vi "Auto_New.vi"() -> ()   [LabVIEW 2017]
uses:
  Control/Saurabh/prosucer_consumer_enum1.ctl
  <vilib>/Utility/error.llb/DialogType.ctl
  <vilib>/addons/database/Connection.llb/DB Tools Open Connec (String).vi
  Global/DATA LOG.vi
  Global/Global 1.vi
  <vilib>/addons/database/NI_Database_API.lvlib
panel:
  out "SHIFT":string
  in  "BARCODE RECIPE":string(combo)
  out "PLC COM.":bool
  out "SHIFT_DATA":string[](array[string])
  out "stop":bool
  out "error out 2":errorcluster
  out "Shift 4":i32
  out "Time Stamp Out":timestamp[](array[timestamp]) format="%<%X>T"
  out "Time Stamp Out 4":timestamp[](array[timestamp]) format="%<%X>T"
  out "Shift_change":bool
  out "appended array":string[][](array[string])
  out "SHIFT_DATA 2":string[](array[string])
  in  "error in (no error)":errorcluster
  in  "Tab Control":enum32{"Screen 1", "Screen 2", "Daignostic"}(tab)
  out "OP 50":bool
  out "OP 40":bool
  out "OP 30":bool
  out "OP - 50":T1 {"RH Motor Screw" format="%#.2g N-m"; "LH Motor Screw" format="%#.2g N-m"; "Nut Torque" format="%#.2g N-m"}
  out "OP - 40":T2 {"Stack Load" format="%.2f kg"; "Dispalcement" format="%#.2g mm"; "LH Screw" format="%#.2g N-m"; "RH Screw" format="%#.2g N-m"}
  out "OP - 30":T3 {"Shaft Press Load" format="%#.2g kg"; "Displacement" format="%#.2g mm"}
  in  "stop 2":bool
  out "OP - 10":T4 {"Leak Rate" format="%#.2g SCCM"}
  in  "SIMULATE INPUT":bool[](array[boolean])=[FALSE, FALSE, FALSE, FALSE]
  out "OP - 20":T5 {"Top Load" format="%#.2g kg"; "Top Displace" format="%#.2g mm"; "Bottom Load" format="%#.2g kg"; "Bottom Displace" format="%#.2g mm"}
  out "OP 10 & 20":bool
  out "OP - 60":T6 {"Screw 6" format="%#.2g N-m"; "Screw 5" format="%#.2g N-m"; "Screw 4" format="%#.2g N-m"; "Screw 3" format="%#.2g N-m"; "Screw 2" format="%#.2g N-m"; "Screw 1" format="%#.2g N-m"}
  out "OP - 70":T7 {"Full Open" format="%#.4g V"; "Full Close" format="%#.4g V"}
  out "OP - 110":cluster{"BARCODE":string}
  out "OP - 80":T8 {"Plug Press Load" format="%#.2f kg"}
  out "OP - 90":T9 {"Steam Leak" format="%#_g sccm"; "Seat Leak" format="%#_g LPM"}
  out "OP - 100":T10 {"Response Time REV" format="%#_g msec"; "Response time FWD" format="%#_g msec"; "Motor Full Open" format="%#.2f V"; "Motor Start Back" format="%#.2f V"; "Motor Full Close" format="%#.2f V"; "Motor Start Of Close" format="%#.2f V"; "Motor Peak" format="%#.2f A"; "Sensor O/P Full Close" format="%#.2f V"; "Sensor O/P Start Of Close" format="%#.2f V"; "Sensor O/P Open" format="%#.2f V"}
  out "OP 60":bool
  out "OP 70 & 80":bool
  out "OP 90 -100 - 110":bool
  out "OP110 STATUS":dbl[](array[numeric])
  out "SCAN OP110":string[](array[string])
  out "OP100 STATUS":dbl[](array[numeric])
  out "SCAN OP100":string[](array[string])
  out "OP50 STATUS":dbl[](array[numeric])
  out "SCAN OP50":string[](array[string])
  out "OP90 STATUS":dbl[](array[numeric])
  out "SCAN OP90":string[](array[string])
  out "OP80 STATUS":dbl[](array[numeric])
  out "SCAN OP80":string[](array[string])
  out "OP70 STATUS":dbl[](array[numeric])
  out "SCAN OP70":string[](array[string])
  out "OP60 STATUS":dbl[](array[numeric])
  out "SCAN OP60":string[](array[string])
  out "OP40 STATUS":dbl[](array[numeric])
  out "SCAN OP40":string[](array[string])
  out "OP30 STATUS":dbl[](array[numeric])
  out "SCAN OP30":string[](array[string])
  out "OP20 STATUS":dbl[](array[numeric])
  out "SCAN OP20":string[](array[string])
  out "OP10 STATUS":dbl[](array[numeric])
  out "SCAN OP10":string[](array[string])
  # "Op10 20\nOp30\nOp 40\nOp50\nOp60\nOp70-80\nOp 90-100-110"
  # "SENSOR MIN VLTG"
  # "OP - 50"
  # "OP - 40"
  # "OP - 30"
  # "OP - 10"
  # "OP - 20"
  # "OP - 60"
  # "OP - 70"
  # "OP - 110"
  # "OP - 80"
  # "OP - 90"
  # "OP - 100"
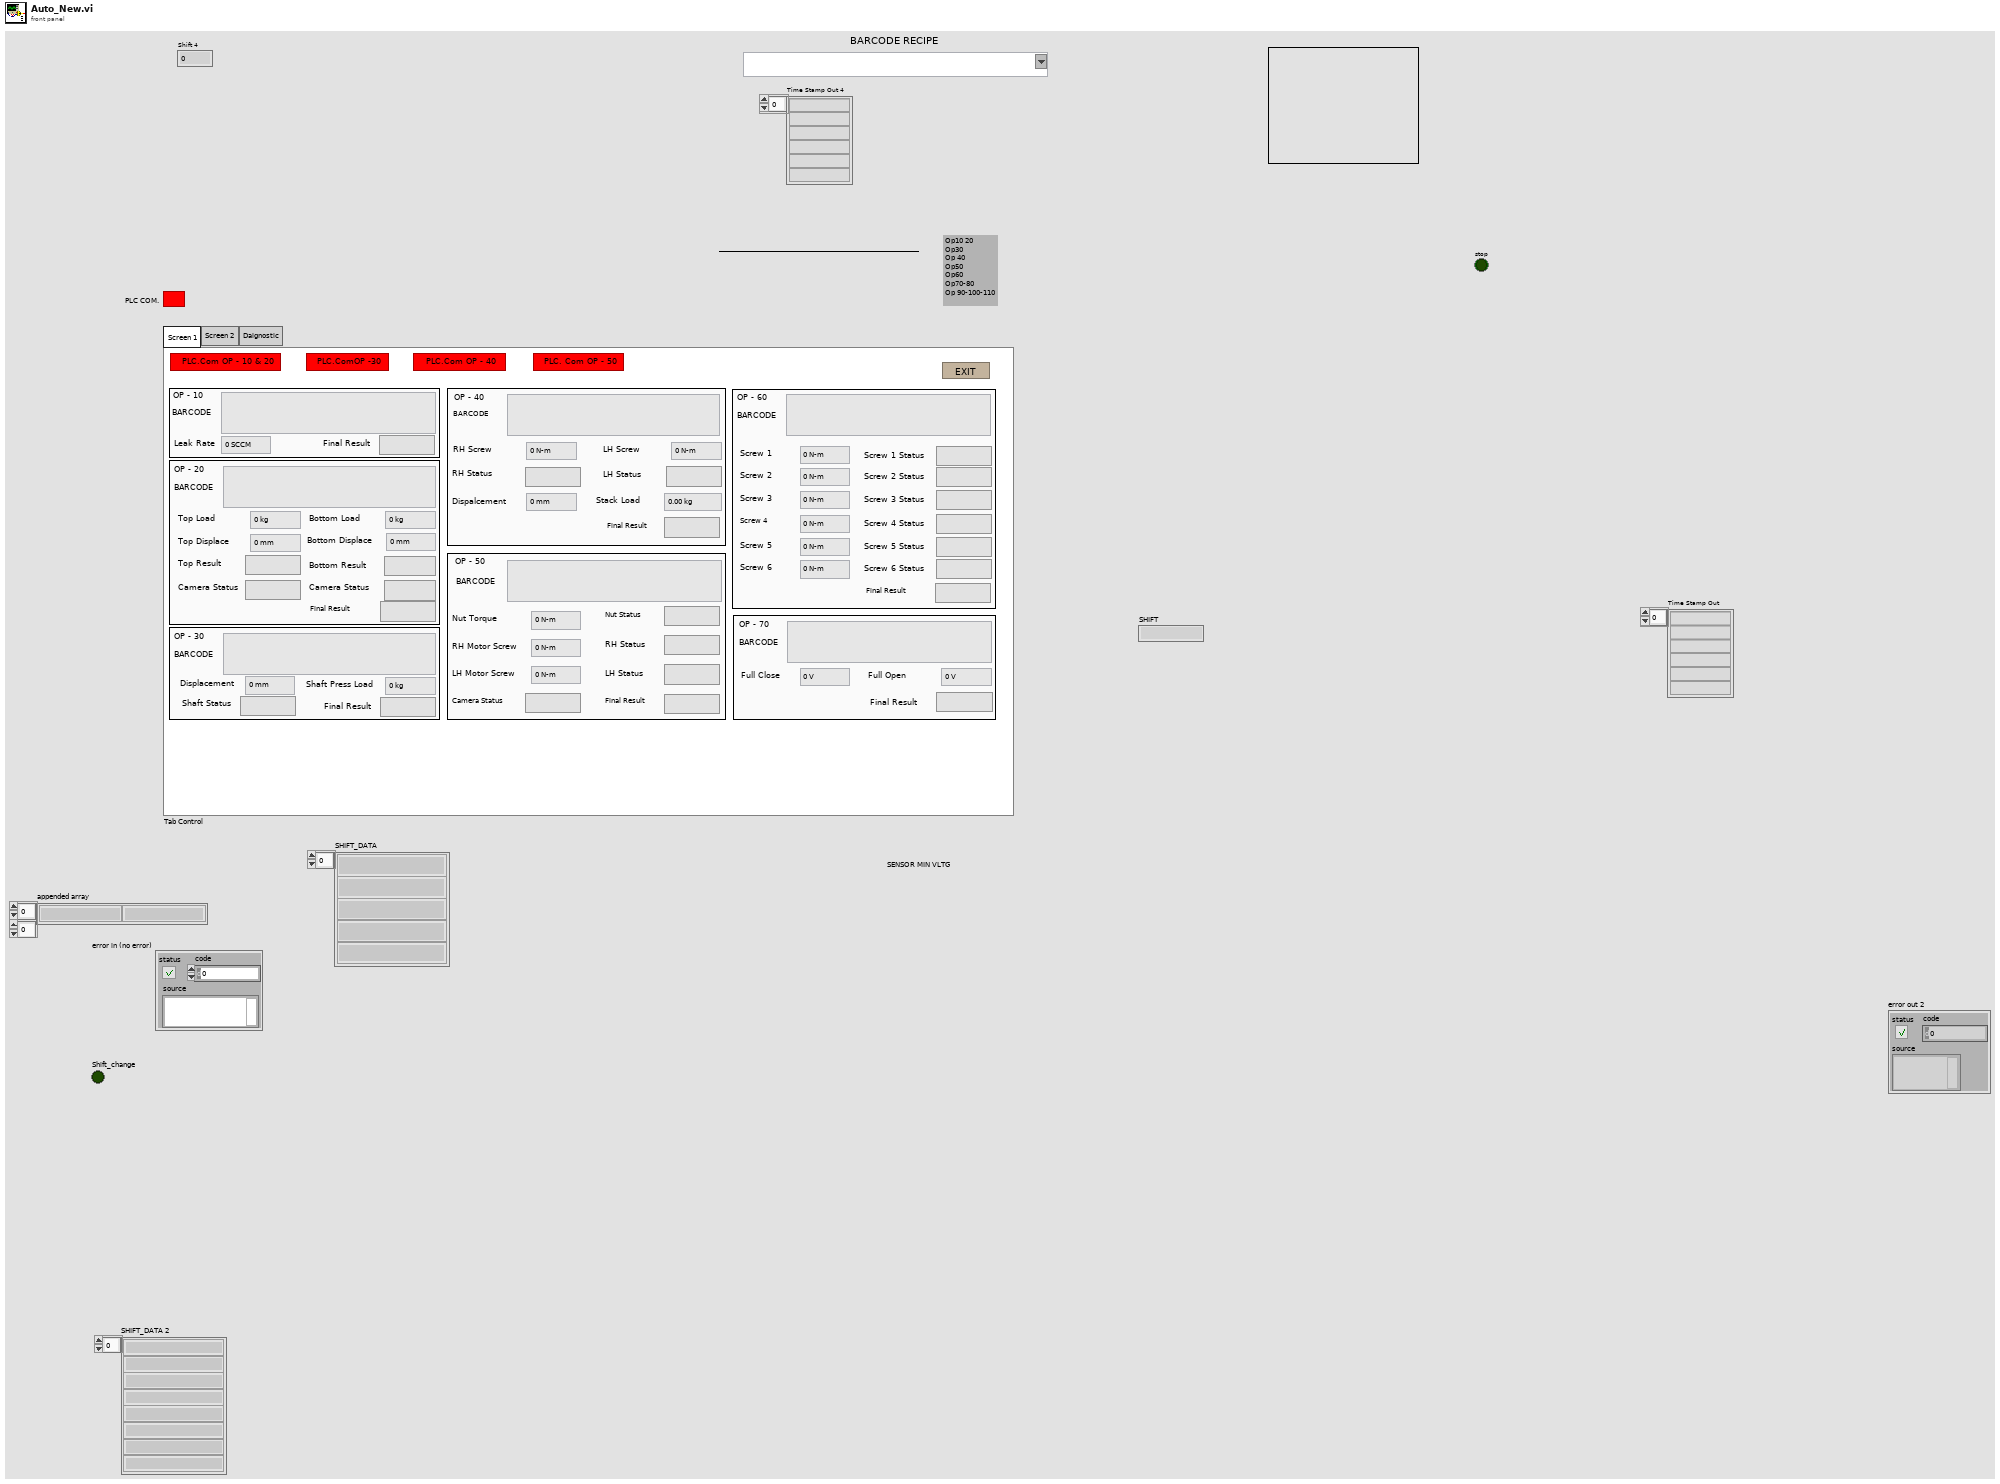
[diagram p1: front panel]
types:
  T1 = cluster{"BARCODE":string, "Nut Torque":dbl, "LH Motor Screw":dbl, "LH Status":bool, "RH Status":bool, "RH Motor Screw":dbl, "Final Result":bool, "Nut Status":bool, "Camera Status":bool}
  T2 = cluster{"BARCODE":string, "RH Screw":dbl, "LH Screw ":dbl, "RH Status":bool, "LH Status":bool, "Dispalcement ":dbl, "Stack Load ":dbl, "Final Result":bool}
  T3 = cluster{"BARCODE":string, "Displacement":dbl, "Shaft Press Load":dbl, "Shaft Status":bool, "Final Result":bool}
  T4 = cluster{"BARCODE":string, "Leak Rate":dbl, "Final Result":bool}
  T5 = cluster{"BARCODE":string, "Bottom Displace":dbl, "Bottom Load":dbl, "Camera Status":bool, "Bottom Result":bool, "Top Displace":dbl, "Top Load ":dbl, "Camera Status":bool, "Top Result":bool, "Final Result":bool}
  T6 = cluster{"BARCODE":string, "Screw 1":dbl, "Screw 2":dbl, "Screw 1 Status":bool, "Screw 2 Status":bool, "Screw 3":dbl, "Final Result":bool, "Screw 3 Status":bool, "Screw 4":dbl, "Screw 5":dbl, "Screw 4 Status":bool, "Screw 5 Status":bool, "Screw 6":dbl, "Screw 6 Status":bool}
  T7 = cluster{"BARCODE":string, "Full Close":dbl, "Full Open":dbl, "Final Result":bool}
  T8 = cluster{"BARCODE":string, "Plug Press Load":dbl, "Final Result":bool, "Loctite Status":bool}
  T9 = cluster{"BARCODE":string, "Seat Leak":dbl, "Seat Status":bool, "Steam Leak":dbl, "Final Result":bool}
  T10 = cluster{"BARCODE":string, "Sensor O/P Open":dbl, "Sensor O/P Start Of Close":dbl, "Final Result":bool, "Sensor O/P Full Close":dbl, "Motor Peak":dbl, "Motor Start Of Close":dbl, "Motor Full Close":dbl, "Motor Start Back":dbl, "Motor Full Open":dbl, "Response time FWD":dbl, "Response Time REV":dbl, "Camera Status":bool}
  T11 = cluster{"OP - 10":cluster{"BARCODE":string, "LEAK RATE":dbl, "RESULT":bool}, "OP - 30":cluster{"BARCODE":string, "Displacement":dbl, "Load":dbl, "Middle Gear Shaft Status":bool, "Final Result":bool}, "OP - 60":cluster{"BARCODE":string, "Screw 1 Data":dbl, "Screw 2 data":dbl, "Screw 1 Status":bool, "Screw 2 Status":bool, "Screw3 Data":dbl, "Final Result":bool, "Screw3 Status":bool, "Screw4 Data":dbl, "Screw5 Data":dbl, "Screw4 Status":bool, "Screw5 Status":bool, "Screw6 Data":dbl, "Screw6 Status":bool}, "OP - 70":cluster{"BARCODE":string, "Sensor MIN Vltg":dbl, "Sensor MAX Vltg":dbl, "Final Result":bool}, "OP - 80":cluster{"BARCODE":string, "Load":dbl, "Final Result":bool, "Dispensing":bool}, "OP - 90":cluster{"BARCODE":string, "Seat LT Data":dbl, "Seat Status":bool, "Steam LT Data":dbl, "Final Result":bool}, "OP - 110":cluster{"BARCODE":string}, "OP - 20":cluster{"BARCODE":string, "Bottom Displace":dbl, "Bottom Load":dbl, "Camera Status":bool, "Bottom Result":bool, "Top Displace":dbl, "Top Load ":dbl, "Camera Status":bool, "Top Result":bool, "Final Result":bool}, "OP - 40":cluster{"BARCODE":string, "RH Screw":dbl, "LH Screw ":dbl, "RH Status":bool, "LH Status":bool, "Dispalcement ":dbl, "Stack Load ":dbl, "Final Result":bool}, "OP - 50":cluster{"BARCODE":string, "Nut Torque":dbl, "LH Motor Screw":dbl, "LH Status":bool, "RH Status":bool, "RH Motor Screw":dbl, "Final Result":bool, "Nut Status":bool, "Camera Status":bool}, "OP - 100":cluster{"BARCODE":string, "Sensor O/P Open":dbl, "Sensor O/P Start Of Close":dbl, "Final Result":bool, "Sensor O/P Full Close":dbl, "Motor Peak":dbl, "Motor Start Of Close":dbl, "Motor Full Close":dbl, "Motor Start Back":dbl, "Motor Full Open":dbl, "Response time FWD":dbl, "Response Time REV":dbl, "Camera Status":bool}}
  T12 = typedef "prosucer_consumer_enum1.ctl" = enum16{"-1", "SCAN1", "SCAN2", "SCAN3", "SCAN4", "SCAN5", "SCAN6", "SCAN7", "SCAN8", "SCAN9", "SCAN10", "SCAN11", "STOP", "DATALOG1", "DATALOG2", "DATALOG3", "DATALOG4", "DATALOG5", "DATALOG6", "DATALOG7", "DATALOG8", "DATALOG9", "DATALOG10", "DATALOG11", "CYCLE_START1", "CYCLE_START2", "CYCLE_START3", "CYCLE_START4", "BARCODE RECIPE", "EMERGENCY STOP"}
  T13 = typedef "NI_Database_API.lvlib/Conn ObjectReference.ctl" = refnum<k1>
  T14 = typedef "OUTPUT Cluster Indicator.ctl" = cluster{"OP - 10":cluster{"BARCODE":string, "LEAK RATE":dbl, "RESULT":bool}, "OP - 30":cluster{"BARCODE":string, "Displacement":dbl, "Load":dbl, "Middle Gear Shaft Status":bool, "Final Result":bool}, "OP - 60":cluster{"BARCODE":string, "Screw 1 Data":dbl, "Screw 2 data":dbl, "Screw 1 Status":bool, "Screw 2 Status":bool, "Screw3 Data":dbl, "Final Result":bool, "Screw3 Status":bool, "Screw4 Data":dbl, "Screw5 Data":dbl, "Screw4 Status":bool, "Screw5 Status":bool, "Screw6 Data":dbl, "Screw6 Status":bool}, "OP - 70":cluster{"BARCODE":string, "Sensor MIN Vltg":dbl, "Sensor MAX Vltg":dbl, "Final Result":bool}, "OP - 80":cluster{"BARCODE":string, "Load":dbl, "Final Result":bool, "Dispensing":bool}, "OP - 90":cluster{"BARCODE":string, "Seat LT Data":dbl, "Seat Status":bool, "Steam LT Data":dbl, "Final Result":bool}, "OP - 110":cluster{"BARCODE":string}, "OP - 20":cluster{"BARCODE":string, "Bottom Displace":dbl, "Bottom Load":dbl, "Camera Status":bool, "Bottom Result":bool, "Top Displace":dbl, "Top Load ":dbl, "Camera Status":bool, "Top Result":bool, "Final Result":bool}, "OP - 40":cluster{"BARCODE":string, "RH Screw":dbl, "LH Screw ":dbl, "RH Status":bool, "LH Status":bool, "Dispalcement ":dbl, "Stack Load ":dbl, "Final Result":bool}, "OP - 50":cluster{"BARCODE":string, "Nut Torque":dbl, "LH Motor Screw":dbl, "LH Status":bool, "RH Status":bool, "RH Motor Screw":dbl, "Final Result":bool, "Nut Status":bool, "Camera Status":bool}, "OP - 100":cluster{"BARCODE":string, "Sensor O/P Open":dbl, "Sensor O/P Start Of Close":dbl, "Final Result":bool, "Sensor O/P Full Close":dbl, "Motor Peak":dbl, "Motor Start Of Close":dbl, "Motor Full Close":dbl, "Motor Start Back":dbl, "Motor Full Open":dbl, "Response time FWD":dbl, "Response Time REV":dbl, "Camera Status":bool}}
  T15 = typedef "DialogType.ctl" = u16
  T16 = cluster{"trimmed string":string, "SHIFT":string, "date/time string":string, string, "Input 2":string}
  T17 = cluster{"SHIFT":string, "date/time string":string, "Input 2":string, string}
  T18 = cluster{"date/time string":string, "Input 2":string, "Input 2":string, "Input 2":string, "Input 2":string, "Input 2":string, "Input 2":string, "Input 2":string, "Input 2":string, "Input 2":string, "Input 2":string}
  T19 = cluster{"date/time string":string, "SHIFT":string, "Input 2":string, "Input 2":string, "Input 2":string, "Input 2":string, "Input 2":string, "Input 2":string, "Input 2":string, "Input 2":string, "Input 2":string, "Input 2":string}
  T20 = cluster{"date/time string":string, "Input 2":string, "Input 2":string, "Input 2":string, "Input 2":string}
  T21 = cluster{"date/time string":string, "SHIFT":string, "Input 2":string, "Input 2":string, "Input 2":string, "Input 2":string}
  T22 = cluster{"date/time string":string, "Input 2":string, "Input 2":string, "Input 2":string, "Input 2":string, "Input 2":string, "Input 2":string, "Input 2":string, "Input 2":string}
  T23 = cluster{"date/time string":string, "SHIFT":string, "Input 2":string, "Input 2":string, "Input 2":string, "Input 2":string, "Input 2":string, "Input 2":string, "Input 2":string, "Input 2":string}
  T24 = cluster{"date/time string":string, "SHIFT":string, "Input 2":string, "Input 2":string, "Input 2":string, "Input 2":string, "Input 2":string, "Input 2":string}
  T25 = cluster{"date/time string":string, "Input 2":string, "Input 2":string, "Input 2":string, "Input 2":string, "Input 2":string, "Input 2":string, "Input 2":string, "Input 2":string, "Input 2":string, "Input 2":string, "Input 2":string, "Input 2":string, "Input 2":string}
  T26 = cluster{"date/time string":string, "SHIFT":string, "Input 2":string, "Input 2":string, "Input 2":string, "Input 2":string, "Input 2":string, "Input 2":string, "Input 2":string, "Input 2":string, "Input 2":string, "Input 2":string, "Input 2":string, "Input 2":string}
  T27 = cluster{"date/time string":string, "Input 2":string, "Input 2":string, "Input 2":string}
  T28 = cluster{"date/time string":string, "SHIFT":string, "Input 2":string, "Input 2":string, "Input 2":string}
  T29 = cluster{"Input 2":string, "SHIFT":string, "date/time string":string, "Input 2":string, "Input 2":string, "Input 2":string}
  T30 = cluster{"BARCODE":string, "Seat LT Data":dbl, "Seat Status":bool, "Steam LT Data":dbl, "Final Result":bool}
  T31 = cluster{"BARCODE":string, "LEAK RATE":dbl, "RESULT":bool}
  T32 = cluster{"BARCODE":string, "Displacement":dbl, "Load":dbl, "Middle Gear Shaft Status":bool, "Final Result":bool}
  T33 = cluster{"BARCODE":string, "Screw 1 Data":dbl, "Screw 2 data":dbl, "Screw 1 Status":bool, "Screw 2 Status":bool, "Screw3 Data":dbl, "Final Result":bool, "Screw3 Status":bool, "Screw4 Data":dbl, "Screw5 Data":dbl, "Screw4 Status":bool, "Screw5 Status":bool, "Screw6 Data":dbl, "Screw6 Status":bool}
  T34 = cluster{"BARCODE":string, "Sensor MIN Vltg":dbl, "Sensor MAX Vltg":dbl, "Final Result":bool}
  T35 = cluster{"BARCODE":string, "Load":dbl, "Final Result":bool, "Dispensing":bool}
  T36 = enum32{"invalid app kind", "Development System", "Run Time System", "Student Edition", "Embedded LabVIEW", "Evaluation", "Custom"}
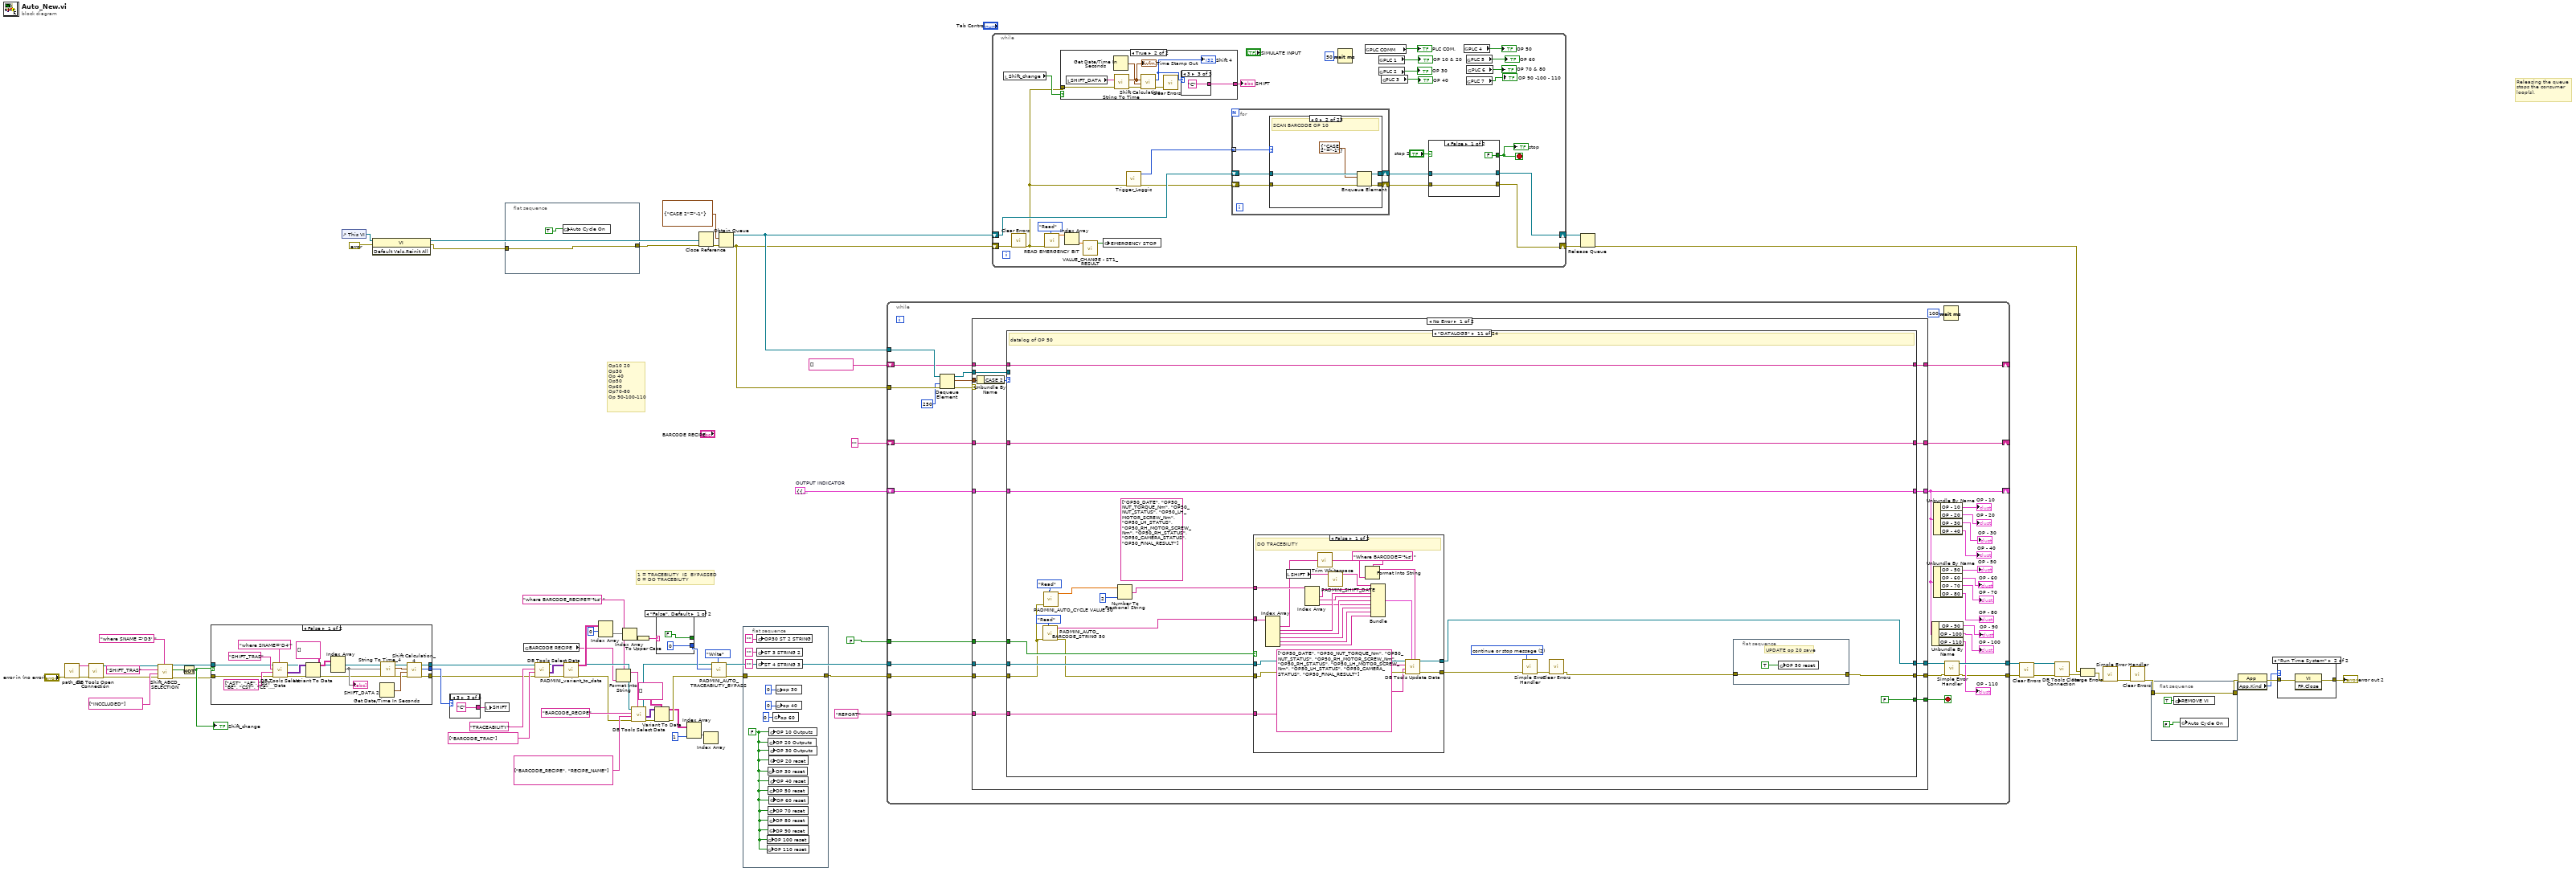
[diagram p0: block diagram]
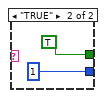
[diagram p2: hidden frame]
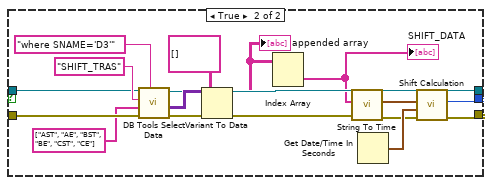
[diagram p3: hidden frame]
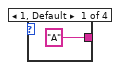
[diagram p4: hidden frame]
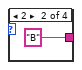
[diagram p5: hidden frame]
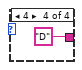
[diagram p6: hidden frame]
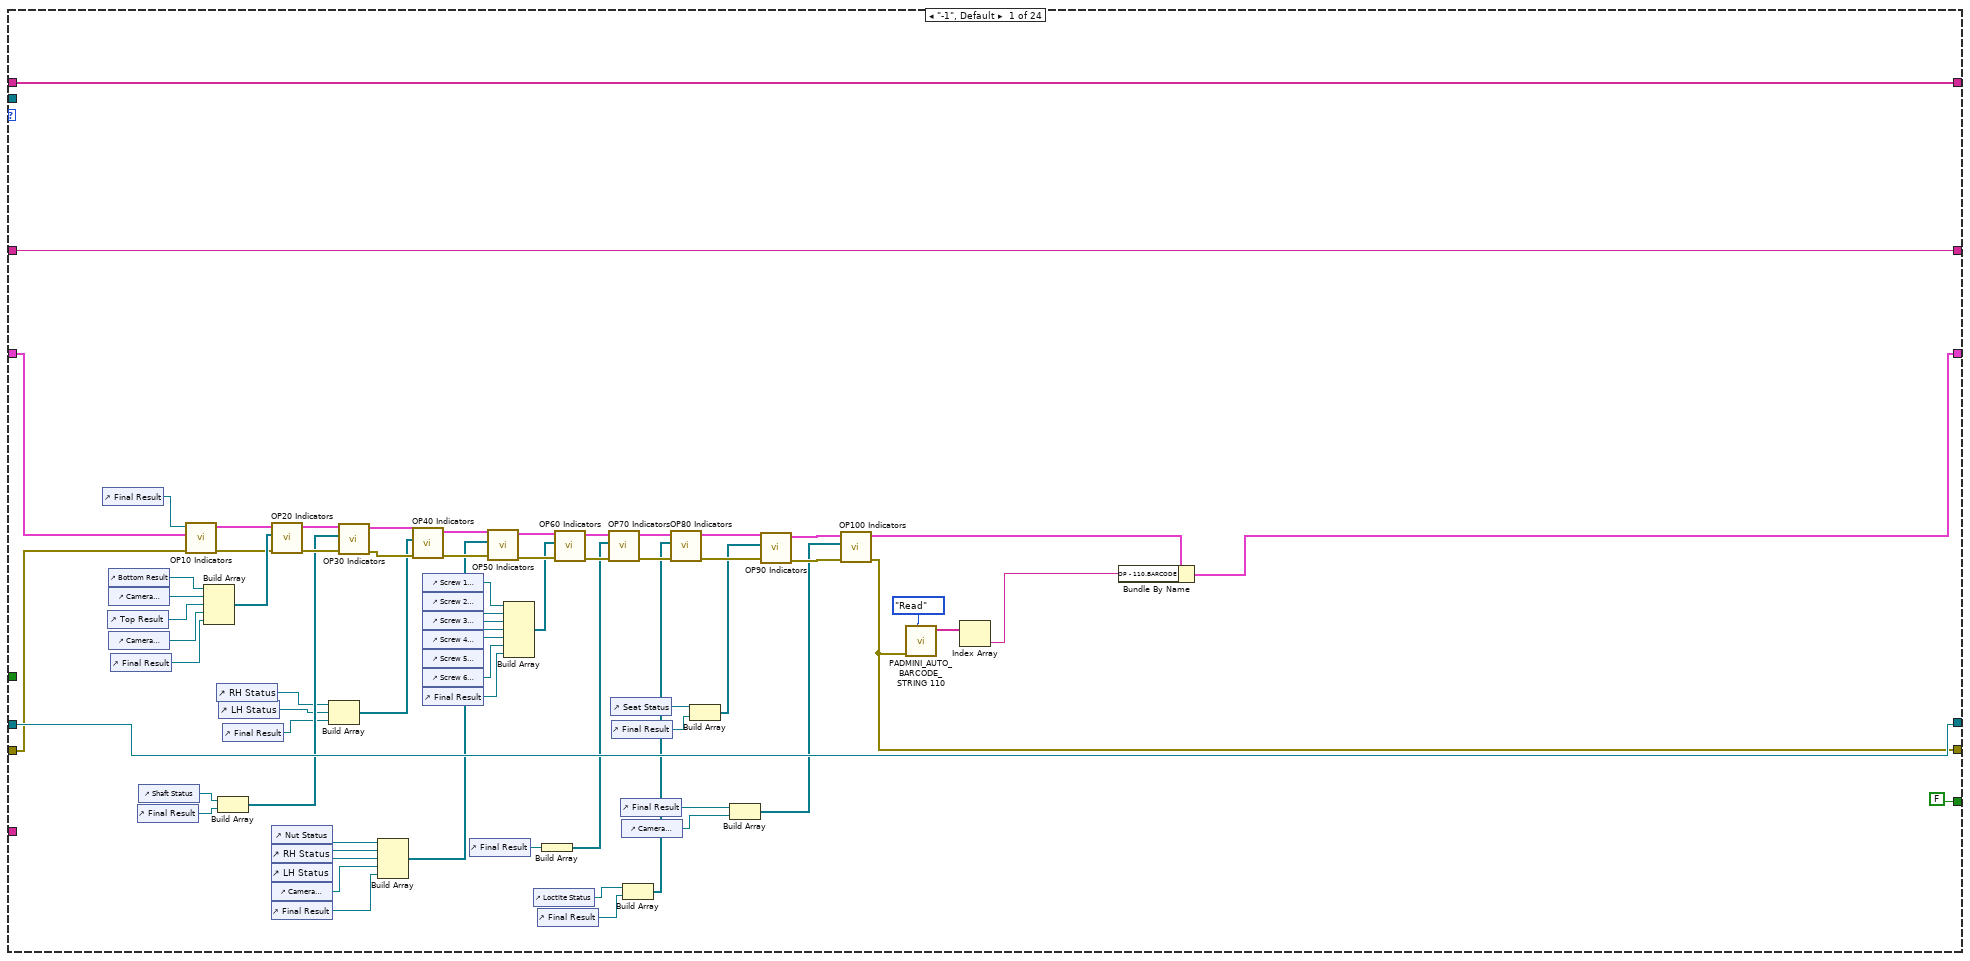
[diagram p7: hidden frame]
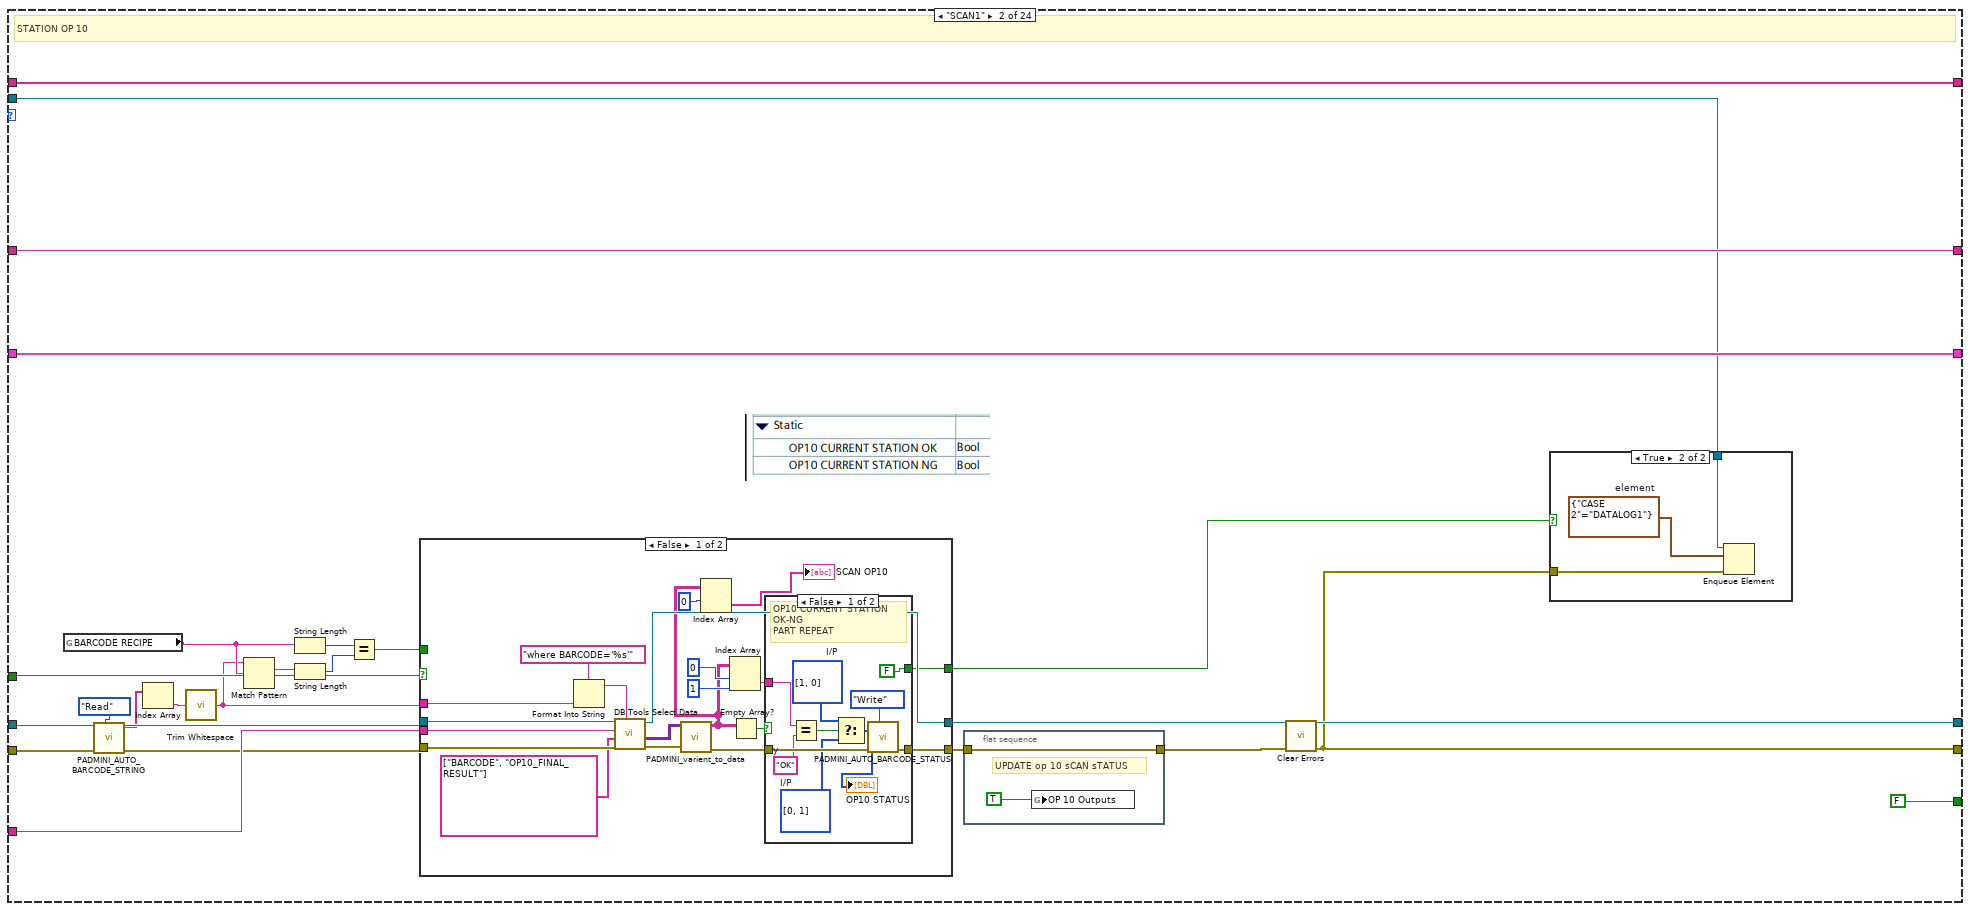
[diagram p8: hidden frame]
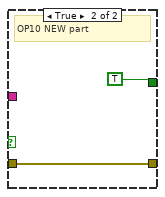
[diagram p10: hidden frame]
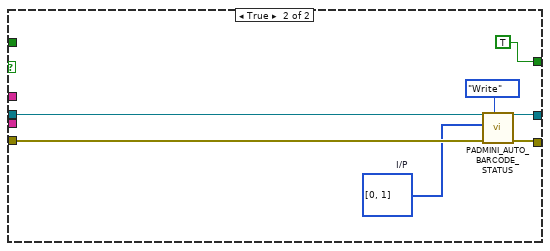
[diagram p11: hidden frame]
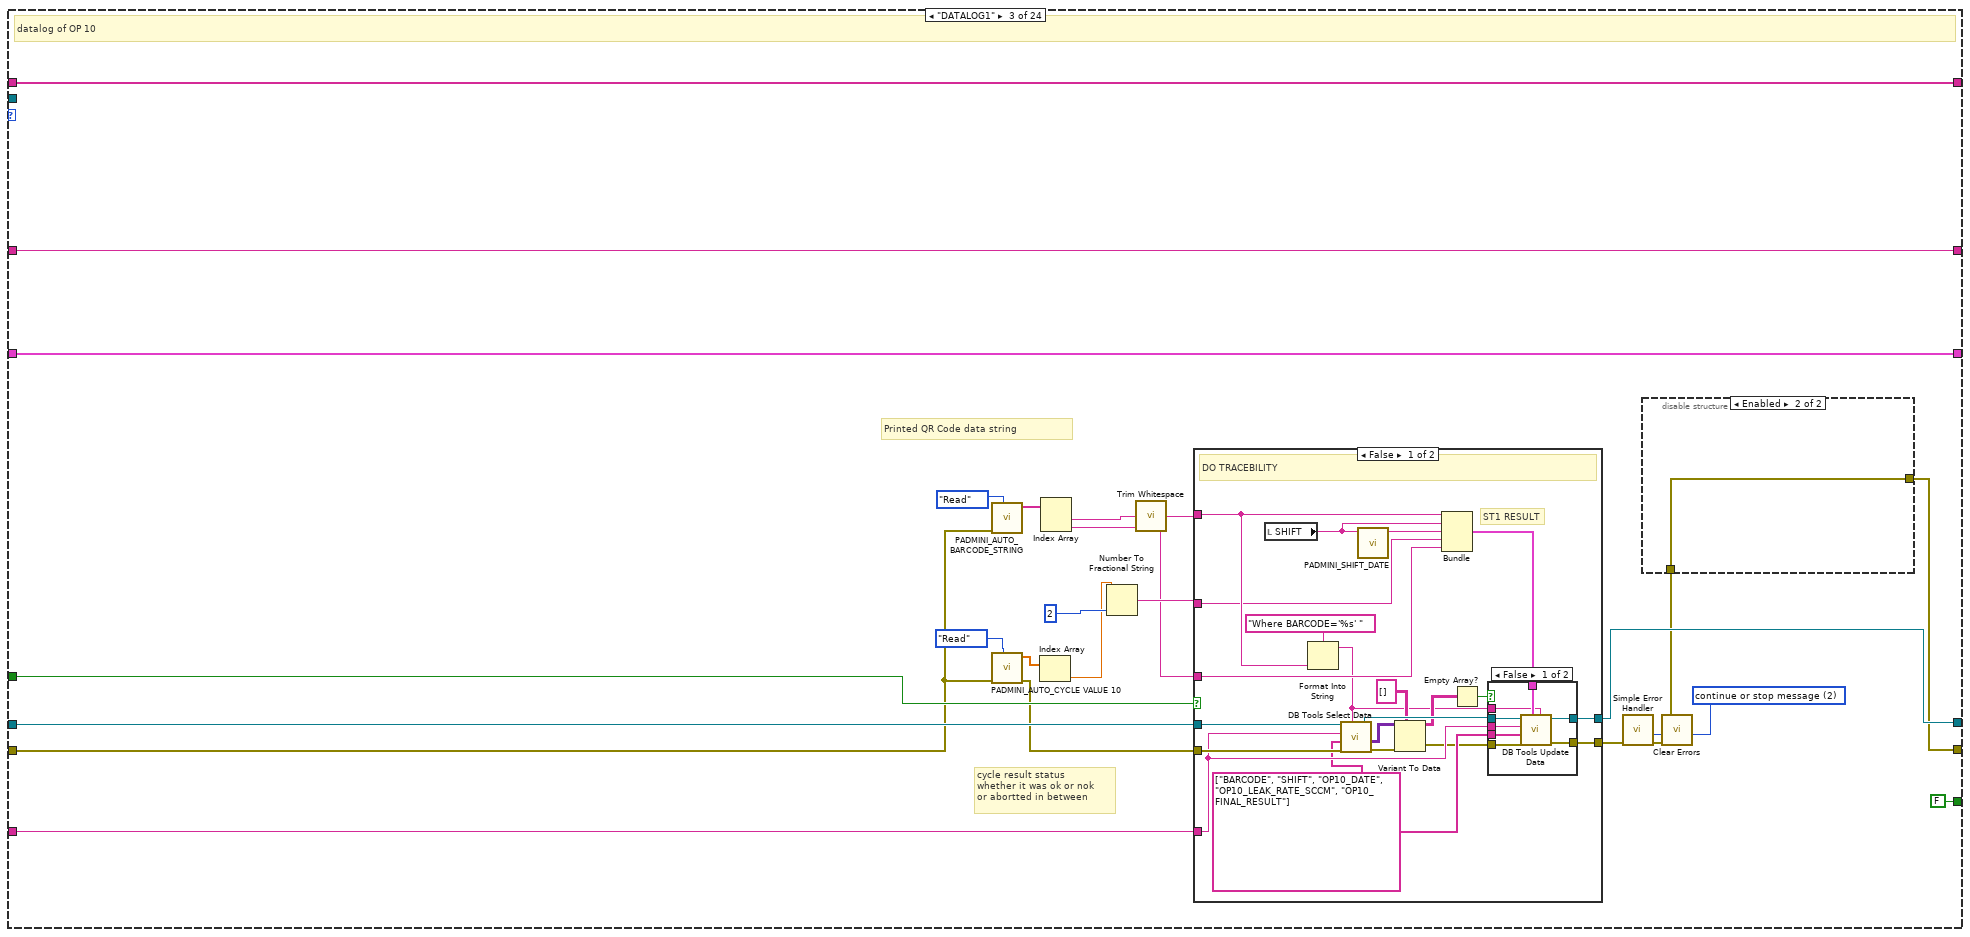
[diagram p12: hidden frame]
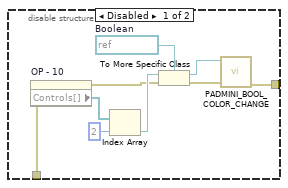
[diagram p13: hidden frame]
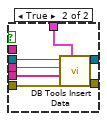
[diagram p14: hidden frame]
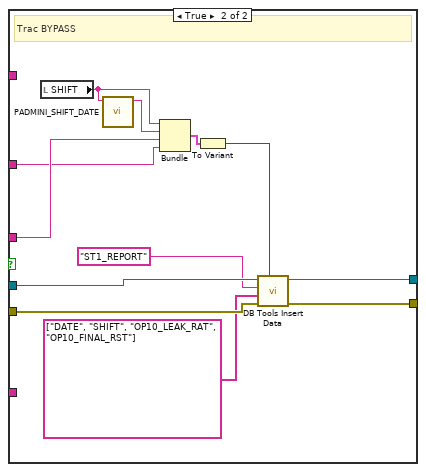
[diagram p15: hidden frame]
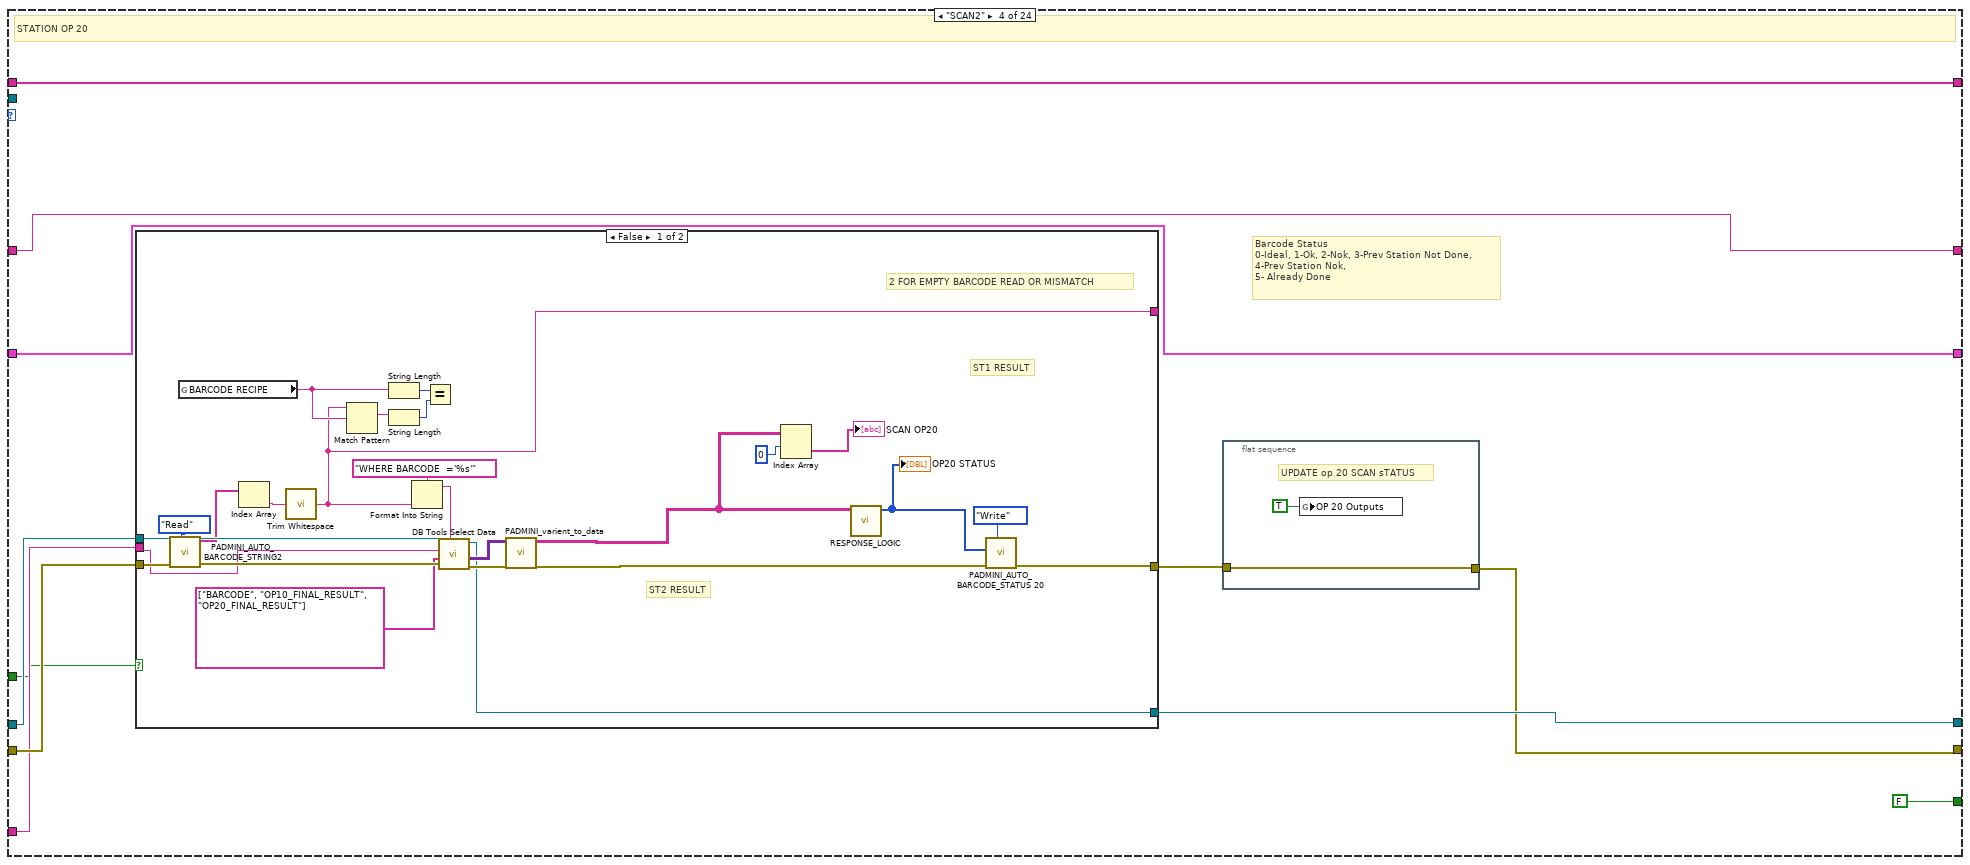
[diagram p16: hidden frame]
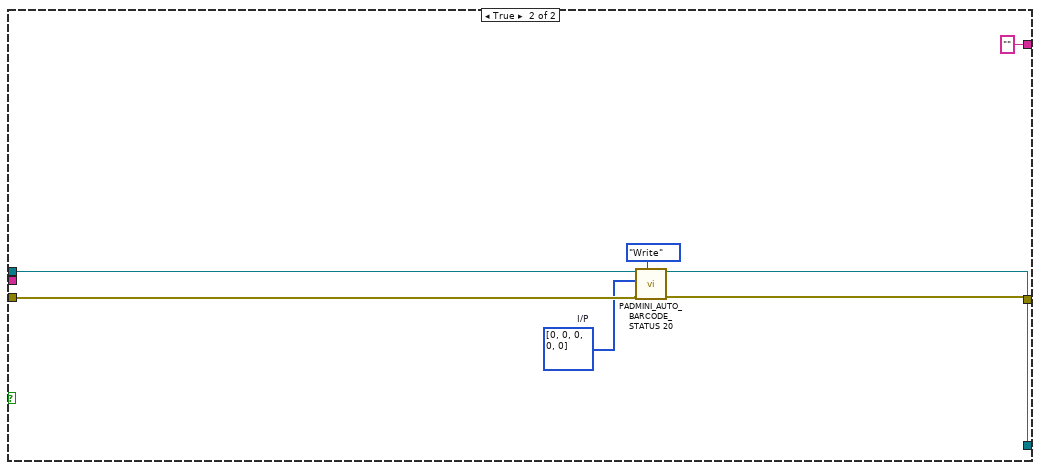
[diagram p17: hidden frame]
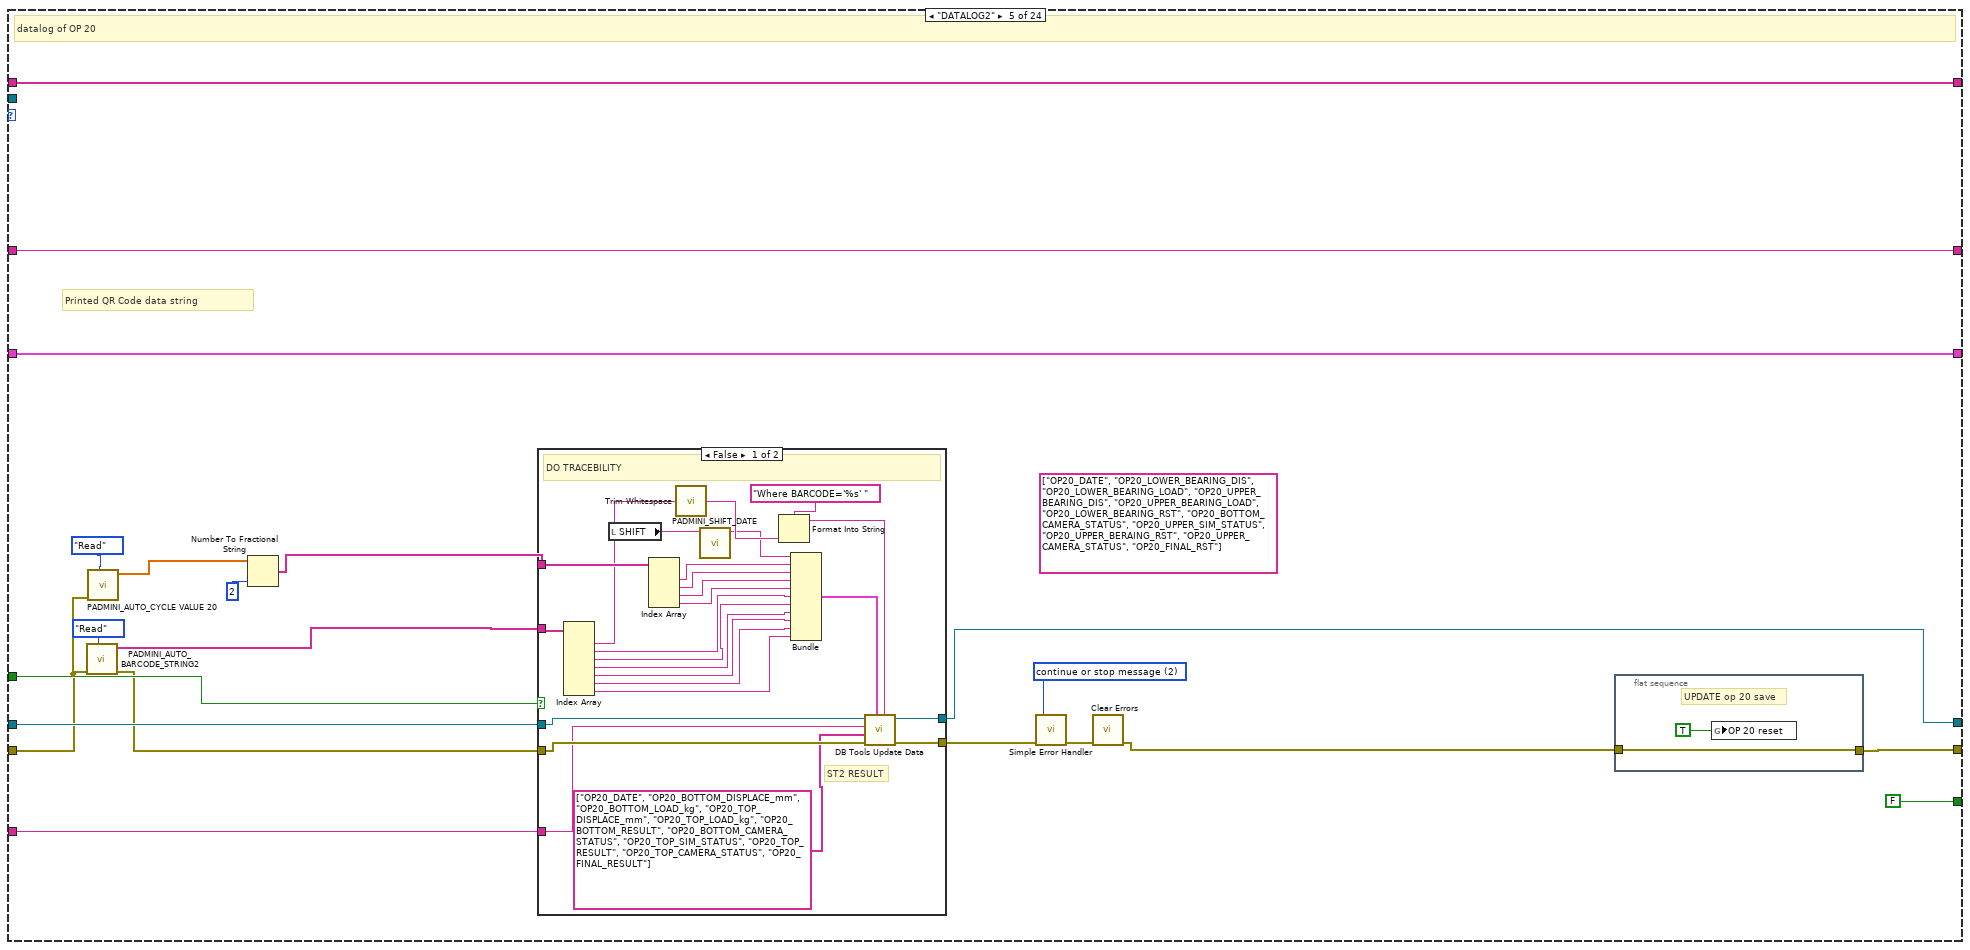
[diagram p18: hidden frame]
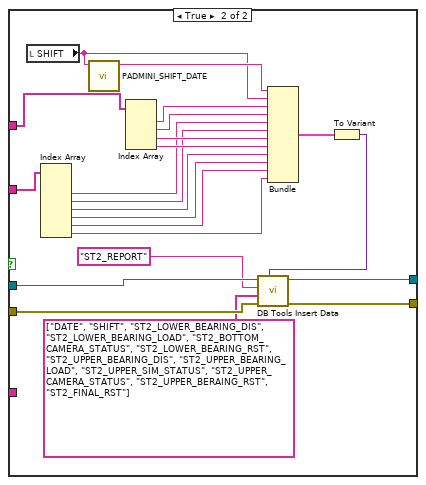
[diagram p19: hidden frame]
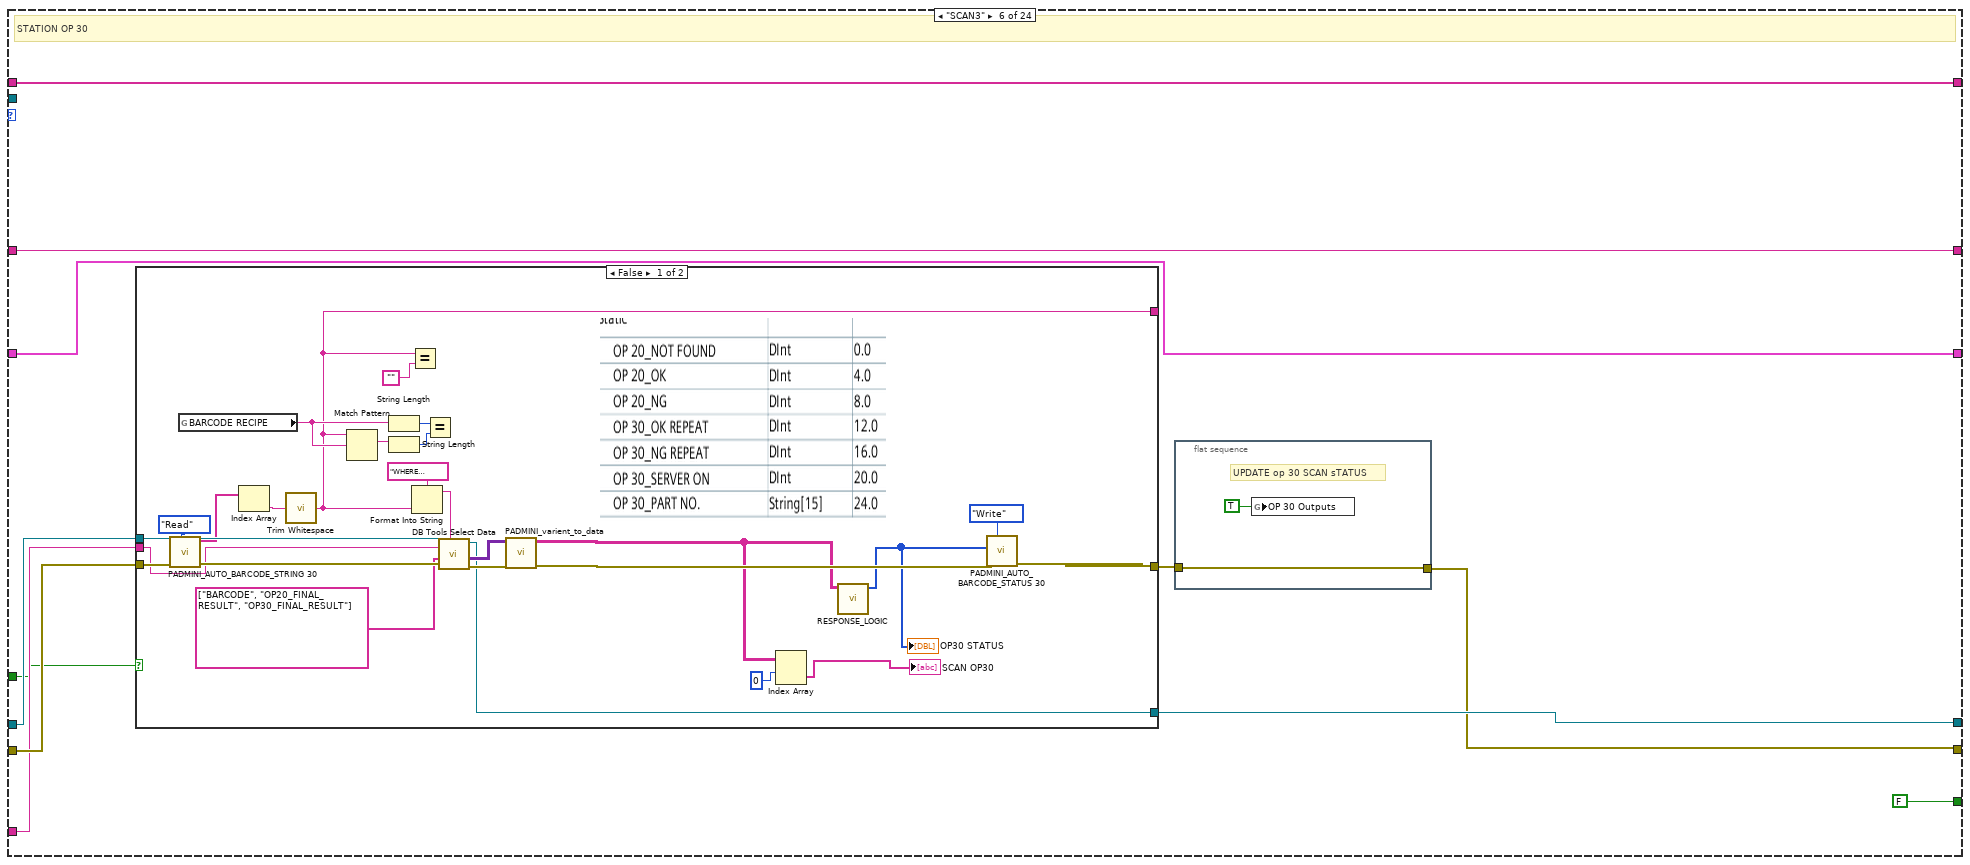
[diagram p20: hidden frame]
diagram:
  w1 = T11 {"OP - 10"={"BARCODE"="", "LEAK RATE"=0.0, "RESULT"=FALSE}, "OP - 30"={"BARCODE"="", "Displacement"=0.0, "Load"=0.0, "Middle Gear Shaft Status"=FALSE, "Final Result"=FALSE}, "OP - 60"={"BARCODE"="", "Screw 1 Data"=0.0, "Screw 2 data"=0.0, "Screw 1 Status"=FALSE, "Screw 2 Status"=FALSE, "Screw3 Data"=0.0, "Final Result"=FALSE, "Screw3 Status"=FALSE, "Screw4 Data"=0.0, "Screw5 Data"=0.0, "Screw4 Status"=FALSE, "Screw5 Status"=FALSE, "Screw6 Data"=0.0, "Screw6 Status"=FALSE}, "OP - 70"={"BARCODE"="", "Sensor MIN Vltg"=0.0, "Sensor MAX Vltg"=0.0, "Final Result"=FALSE}, "OP - 80"={"BARCODE"="", "Load"=0.0, "Final Result"=FALSE, "Dispensing"=FALSE}, "OP - 90"={"BARCODE"="", "Seat LT Data"=0.0, "Seat Status"=FALSE, "Steam LT Data"=0.0, "Final Result"=FALSE}, "OP - 110"={"BARCODE"=""}, "OP - 20"={"BARCODE"="", "Bottom Displace"=0.0, "Bottom Load"=0.0, "Camera Status"=FALSE, "Bottom Result"=TRUE, "Top Displace"=0.0, "Top Load "=0.0, "Camera Status"=FALSE, "Top Result"=FALSE, "Final Result"=FALSE}, "OP - 40"={"BARCODE"="", "RH Screw"=0.0, "LH Screw "=0.0, "RH Status"=FALSE, "LH Status"=FALSE, "Dispalcement "=0.0, "Stack Load "=0.0, "Final Result"=FALSE}, "OP - 50"={"BARCODE"="", "Nut Torque"=0.0, "LH Motor Screw"=0.0, "LH Status"=FALSE, "RH Status"=FALSE, "RH Motor Screw"=0.0, "Final Result"=FALSE, "Nut Status"=FALSE, "Camera Status"=FALSE}, "OP - 100"={"BARCODE"="", "Sensor O/P Open"=0.0, "Sensor O/P Start Of Close"=0.0, "Final Result"=FALSE, "Sensor O/P Full Close"=0.0, "Motor Peak"=0.0, "Motor Start Of Close"=0.0, "Motor Full Close"=0.0, "Motor Start Back"=0.0, "Motor Full Open"=0.0, "Response time FWD"=0.0, "Response Time REV"=0.0, "Camera Status"=FALSE}}  # OUTPUT INDICATOR
  # "Op10 20\nOp30\nOp 40\nOp50\nOp60\nOp70-80\nOp 90-100-110"
  # "1 = TRACEBILITY  IS  BYPASSED\n0 = DO TRACEBILITY"
  # "Releasing the queue stops the consumer loop(s)."
  n1 = call "path_db.vi"("error in"="error in (no error)") -> ("error out"=w48:errorcluster, "resulting string"=w69:string)  [unwired: 9 in]
  n2 = call-poly <vilib>:"DB Tools Open Connection.vi"("error in (no error)"=w48, "connection information"=w69) -> ("error out"=w47:errorcluster, "connection reference"=w41:T13)  [unwired: 6 in]
  n3 = call "Shift_ABCD_SELECTION.vi"("Where"="where SNAME ='D3' ", "error in (no error)"=w47, "Array"=string[] ["INCCLUDED"], "table"="SHIFT_TRAS", "Refnum in"=w41) -> ("error out"=w5:errorcluster, "Boolean"=w60:bool, "Refnum out"=w61:T13)  [unwired: 4 in]
  n4 = Not(x=w60) -> (.not. x?=w59:bool)
  "Shift_change" <- w59
  n5 = case shown="False" w59 {
    tunnel: [w74 w98] -> w65
    tunnel: w61 -> [w77 w96]
    tunnel: w5 -> [w76 w95]
    tunnel: [w75 w94] -> w30
    tunnel: [w73 w88] -> w29
    frame False {
      n6 = call <vilib>:"DB Tools Select Data.vi"("condition"="where SNAME='D4'", "error in (no error)"=w76, "columns"=string[] ["AST", "AE", "BST", "BE", "CST", "CE", "DST", "DE"], "table"="SHIFT_TRAS", "connection reference"=w77) -> ("error out"=w83:errorcluster, "data"=w87:variant[][], "connection reference out"=w75:T13)  [unwired: 1 in]
      n7 = Variant To Data(error in=w83, type=string[][] [], Variant=w87) -> (data=w80:string[][], error out=w73:errorcluster)
      n8 = Index Array(array=w80) -> (element=w79:string[])  [unwired: 2 in]
      "SHIFT_DATA 2" <- w79
      n9 = Get Date/Time In Seconds() -> (seconds since 1Jan1904=w82:timestamp)
      n10 = call "String To Time_4.vi"("String Array In"=w79) -> ("Time Stamp Out"=w78:timestamp[])  [unwired: 9 in, 1 out]
      n11 = call "Shift Calculation_4.vi"("Current Time"=w82, "Time Stamp Out"=w78) -> ("Shift"=w74:i32)  [unwired: 8 in, 1 out]
    }
    frame True {
      n12 = call <vilib>:"DB Tools Select Data.vi"("condition"="where SNAME='D3'", "error in (no error)"=w95, "columns"=string[] ["AST", "AE", "BST", "BE", "CST", "CE"], "table"="SHIFT_TRAS", "connection reference"=w96) -> ("error out"=w100:errorcluster, "data"=w104:variant[][], "connection reference out"=w94:T13)  [unwired: 1 in]
      n13 = Variant To Data(error in=w100, type=string[][] [], Variant=w104) -> (data=w92:string[][], error out=w90:errorcluster)
      "appended array" <- w92
      n14 = Index Array(array=w92) -> (element=w91:string[])  [unwired: 2 in]
      "SHIFT_DATA" <- w91
      n15 = call "String To Time.vi"("error in (no error)"=w90, "String Array In"=w91) -> ("error out"=w89:errorcluster, "Time Stamp Out"=w97:timestamp[])  [unwired: 8 in]
      n16 = Get Date/Time In Seconds() -> (seconds since 1Jan1904=w99:timestamp)
      n17 = call "Shift Calculation.vi"("error in (no error)"=w89, "Current Time"=w99, "Time Stamp Out"=w97) -> ("error out"=w88:errorcluster, "Shift"=w98:i32)  [unwired: 7 in]
    }
  }
  n18 = control-ref of="This VI"() -> (w45:refnum<vi>)
  n19 = invoke class="VI" method="Default Vals.Reinit All"(reference=w45, error in=errorcluster {"status"=FALSE, "code"=0, "source"=""} ("error in (no error)")) -> (reference out=w44:refnum<vi>, error out=w2:errorcluster)  [unwired: 1 in, 1 out]
  n20 = case shown="3" w65 {
    tunnel: ["A" "B" "C" "D"] -> w58
    frame 1, Default {
    }
    frame 2 {
    }
    frame 3 {
    }
    frame 4 {
    }
  }
  n21 = local write "SHIFT"(w58) -> ()
  n22 = flat-sequence {
    tunnel: [w110] -> w3
    tunnel: w2 -> [w110]
    frame #0 {
      n23 = global write "DATA LOG.vi" "Auto Cycle On"(TRUE) -> ()
    }
  }
  n24 = global read "Global 1.vi" "BARCODE RECIPE"() -> (w11:string)
  n25 = call <vilib>:"DB Tools Select Data.vi"("error in (no error)"=w29, "columns"=string[] ["BARCODE_TRAC"], "table"="TRACEABILITY", "connection reference"=w30) -> ("error out"=w39:errorcluster, "data"=w38:variant[][], "connection reference out"=w17:T13)  [unwired: 2 in]
  n26 = call "PADMINI_varient_to_data.vi"("error in (no error)"=w39, "data"=w38) -> ("error out"=w15:errorcluster, "Array"=w37:string[][])  [unwired: 8 in]
  n27 = Index Array(array=w37, index (row)=0 ("disabled index (col)")) -> (element=w36:string[])  [unwired: 1 in]
  n28 = Format Into String(format string="where BARCODE_RECIPE='%s' ", w11) -> (resulting string=w9:string)  [unwired: 2 in, 1 out]
  n29 = Index Array(array=w36) -> (element=w32:string)  [unwired: 1 in]
  n30 = call <vilib>:"DB Tools Select Data.vi"("condition"=w9, "error in (no error)"=w15, "columns"=string[] ["BARCODE_RECIPE", "RECIPE_NAME"], "table"="BARCODE_RECIPE", "connection reference"=w17) -> ("error out"=w19:errorcluster, "data"=w18:variant[][], "connection reference out"=w16:T13)  [unwired: 1 in]
  n31 = To Upper Case(1:w32) -> (0:w31:string)
  n32 = Variant To Data(error in=w19, type=string[][] [], Variant=w18) -> (data=w12:string[][], error out=w14:errorcluster)
  n33 = case shown="\"False\", Default" w31 {
    tunnel: [FALSE ("BARCODE TRACEABILITY") TRUE ("BARCODE TRACEABILITY")] -> _
    tunnel: [0 1] -> w27
    frame "False", Default {
    }
    frame "TRUE" {
    }
  }
  n34 = Index Array(array=w12, index (col)=1 ("disabled index (col)")) -> (element=w7:string[])  [unwired: 1 in]
  n35 = Close Reference(reference=w44, error in (no error)=w3) -> (error out=w42:errorcluster)
  n36 = Index Array(array=w7) -> ()  [unwired: 1 in, 1 out]
  n37 = call "PADMINI_AUTO_TRACEABILITY_BYPASS.vi"("Enum"=enum16{"Read", "Write"}."Write", "error in (no error)"=w14, "I/P"=w27) -> ("error out"=w25:errorcluster)  [unwired: 7 in, 1 out]
  n38 = Obtain Queue(element data type=cluster{"CASE 2":T12} {"CASE 2"=enum."-1"}, error in (no error)=w42) -> (queue out=w70:refnum<queue>, error out=w22:errorcluster)  [unwired: 3 in, 1 out]
  n39 = flat-sequence {
    tunnel: w25 -> [w119]
    tunnel: [w119] -> w24
    frame #0 {
      w115 = FALSE
      n40 = global write "DATA LOG.vi" "OP30 ST 2 STRING"("" ("OP30 ST 2 STRING")) -> ()
      n41 = global write "DATA LOG.vi" "ST 3 STRING 2"("" ("ST 3 STRING 2")) -> ()
      n42 = global write "DATA LOG.vi" "ST 4 STRING 3"("" ("ST 4 STRING 3")) -> ()
      n43 = global write "DATA LOG.vi" "OP 100 reset"(w115) -> ()
      n44 = global write "DATA LOG.vi" "OP 110 reset"(w115) -> ()
      n45 = global write "DATA LOG.vi" "OP 30 reset"(w115) -> ()
      n46 = global write "DATA LOG.vi" "OP 20 Outputs"(w115) -> ()
      n47 = global write "DATA LOG.vi" "OP 50 reset"(w115) -> ()
      n48 = global write "DATA LOG.vi" "OP 70 reset"(w115) -> ()
      n49 = global write "DATA LOG.vi" "OP 80 reset"(w115) -> ()
      n50 = global write "DATA LOG.vi" "OP 90 reset"(w115) -> ()
      n51 = global write "DATA LOG.vi" "OP 10 Outputs"(w115) -> ()
      n52 = global write "DATA LOG.vi" "OP 30 Outputs"(w115) -> ()
      n53 = global write "DATA LOG.vi" "OP 20 reset"(w115) -> ()
      n54 = global write "DATA LOG.vi" "OP 40 reset"(w115) -> ()
      n55 = global write "DATA LOG.vi" "OP 60 reset"(w115) -> ()
      n56 = global write "DATA LOG.vi" "op 60"(0 ("op 30")) -> ()
      n57 = global write "DATA LOG.vi" "op 30"(0 ("op 30")) -> ()
      n58 = global write "DATA LOG.vi" "op 40"(0 ("op 30")) -> ()
    }
  }
  n59 = while {
    tunnel: w70 -> [w154]
    tunnel: w22 -> [w150]
    tunnel: w24 -> [w149]
    tunnel: w16 -> [w148]
    tunnel: [w123] -> w68
    tunnel: [w147] -> w67
    tunnel: FALSE -> [w146]
    tunnel: "REPORT" -> [w145]
    shift-right: [w143] -> _
    shift-left: string[] [] -> [w144]
    shift-right: [w142] -> _
    shift-left: "" ("trimmed string") -> [w141]
    shift-right: [w130] -> _
    shift-left: w1 -> [w139]
    stop <- w151 stop-if-true
    n60 = Dequeue Element(queue=w154, timeout in ms (-1)=250, error in (no error)=w150) -> (queue out=w126:refnum<queue>, element=w152:cluster{"CASE 2":T12}, error out=w153:errorcluster)  [unwired: 1 out]
    n61 = case shown="No Error" w153 {
      tunnel: w152 -> [w170 _]
      tunnel: [w166 TRUE] -> w151
      tunnel: w149 -> [w167 w1405]
      tunnel: w148 -> [w168 w1404]
      tunnel: [w164 w1405] -> w124
      tunnel: [w165 w1404] -> w147
      tunnel: w146 -> [w163 _]
      tunnel: w145 -> [w162 _]
      tunnel: w144 -> [w161 w1403]
      tunnel: [w160 w1403] -> w143
      tunnel: [w159 w1402] -> w142
      tunnel: w141 -> [w158 w1402]
      tunnel: w139 -> [w157 w1401]
      tunnel: [w156 w1401] -> w130
      tunnel: w126 -> [w155 _]
      frame No Error {
        n62 = Unbundle By Name(w170) -> ("CASE 2"=w169:T12)
        n63 = case shown="\"DATALOG5\"" w169 {
          tunnel: w168 -> [w238 w262 w330 w400 w453 w514 w568 w617 w666 w723 w772 w827 w876 w942 w988 w1035 w1084 w1132 w1181 w1230 w1270 w1329 w1388 w1396]
          tunnel: w167 -> [w235 w258 w307 w399 w440 w513 w554 w616 w652 w722 w759 w826 w862 w941 w977 w1034 w1071 w1131 w1167 w1229 w1269 w1311 w1387 w1398]
          tunnel: [FALSE FALSE FALSE FALSE FALSE FALSE FALSE FALSE FALSE FALSE FALSE FALSE FALSE FALSE FALSE FALSE FALSE FALSE FALSE FALSE FALSE FALSE FALSE TRUE] -> w166
          tunnel: [w238 w260 w327 w397 w450 w511 w565 w614 w663 w720 w769 w824 w873 w939 w985 w1032 w1082 w1129 w1178 w1227 w1267 w1326 w1388 w1395] -> w165
          tunnel: [w172 w240 w326 w394 w435 w508 w549 w611 w647 w717 w754 w821 w857 w936 w972 w1029 w1066 w1126 w1162 w1224 w1264 w1310 w1387 w1397] -> w164
          tunnel: w163 -> [_ w255 w329 w396 w452 w510 w567 w613 w665 w719 w771 w823 w875 w938 w987 w1031 w1065 w1128 w1180 w1226 w1266 w1328 _ _]
          tunnel: w162 -> [_ w261 w328 w398 w451 w512 w566 w615 w664 w721 w770 w825 w874 w940 w986 w1033 w1083 w1130 w1179 w1228 w1268 w1327 _ _]
          tunnel: w161 -> [w237 w259 w323 w391 w449 w506 w564 w609 w662 w715 w768 w819 w872 w934 w984 w1027 w1081 w1124 w1177 w1222 w1262 w1325 w1385 w1399]
          tunnel: [w237 w259 w323 w391 w449 w506 w564 w609 w662 w715 w768 w819 w872 w934 w984 w1027 w1081 w1124 w1177 w1222 w1262 w1325 w1385 w1399] -> w160
          tunnel: [w236 w254 w319 w392 w445 w505 w560 w608 w658 w714 w764 w818 w868 w933 w982 w1026 w1077 w1123 w1173 w1221 w1261 w1321 w1384 w1390] -> w159
          tunnel: w158 -> [w236 w254 w319 w392 w445 w505 w560 w608 w658 w714 w764 w818 w868 w933 w982 w1026 w1077 w1123 w1173 w1221 w1261 w1321 w1384 w1390]
          tunnel: w157 -> [w234 w248 w317 w390 w434 w504 w558 w607 w656 w713 w753 w817 w866 w932 w981 w1025 w1075 w1122 w1171 w1220 w1260 w1319 w1383 w1389]
          tunnel: [w176 w248 w317 w390 w434 w504 w558 w607 w656 w713 w753 w817 w866 w932 w981 w1025 w1075 w1122 w1171 w1220 w1260 w1319 w1383 w1389] -> w156
          tunnel: w155 -> [_ w242 _ _ _ _ _ _ _ _ _ _ _ _ _ _ _ _ _ _ _ _ _ _]
          frame "-1", Default {
            n64 = control-ref of="Final Result"() -> (w225:refnum<vi>)
            n65 = control-ref of="Top Result"() -> (w229:refnum<vi>)
            n66 = control-ref of="Bottom Result"() -> (w231:refnum<vi>)
            n67 = control-ref of="Camera Status"() -> (w230:refnum<vi>)
            n68 = control-ref of="Camera Status"() -> (w228:refnum<vi>)
            n69 = control-ref of="Final Result"() -> (w227:refnum<vi>)
            n70 = control-ref of="Final Result"() -> (w221:refnum<vi>)
            n71 = control-ref of="Shaft Status"() -> (w222:refnum<vi>)
            n72 = call "OP10 Indicators.vi"("error in (no error)"=w235, "OUTPUT INDICATOR"=w234, "Boolean in"=w225) -> ("error out"=w224:errorcluster, "OUTPUT INDICATOR"=w233:T14)  [unwired: 7 in]
            n73 = Build Array(w231, w230, w229, w228, w227) -> (w226:refnum<vi>[])
            n74 = control-ref of="RH Status"() -> (w217:refnum<vi>)
            n75 = Build Array(w222, w221) -> (w220:refnum<vi>[])
            n76 = control-ref of="LH Status"() -> (w216:refnum<vi>)
            n77 = control-ref of="Final Result"() -> (w215:refnum<vi>)
            n78 = call "OP20 Indicators.vi"("error in (no error)"=w224, "Array"=w226, "OUTPUT INDICATOR"=w233) -> ("error out"=w223:errorcluster, "OUTPUT INDICATOR"=w232:T14)  [unwired: 7 in]
            n79 = control-ref of="Nut Status"() -> (w211:refnum<vi>)
            n80 = control-ref of="RH Status"() -> (w210:refnum<vi>)
            n81 = control-ref of="LH Status"() -> (w209:refnum<vi>)
            n82 = control-ref of="Camera Status"() -> (w208:refnum<vi>)
            n83 = control-ref of="Final Result"() -> (w207:refnum<vi>)
            n84 = Build Array(w217, w216, w215) -> (w214:refnum<vi>[])
            n85 = call "OP30 Indicators.vi"("error in (no error)"=w223, "Array"=w220, "OUTPUT INDICATOR"=w232) -> ("error out"=w218:errorcluster, "OUTPUT INDICATOR"=w219:T14)  [unwired: 7 in]
            n86 = Build Array(w211, w210, w209, w208, w207) -> (w206:refnum<vi>[])
            n87 = call "OP40 Indicators.vi"("error in (no error)"=w218, "Array"=w214, "OUTPUT INDICATOR"=w219) -> ("error out"=w213:errorcluster, "OUTPUT INDICATOR"=w212:T14)  [unwired: 7 in]
            n88 = control-ref of="Screw 1 Status"() -> (w202:refnum<vi>)
            n89 = control-ref of="Screw 2 Status"() -> (w201:refnum<vi>)
            n90 = control-ref of="Screw 3 Status"() -> (w200:refnum<vi>)
            n91 = control-ref of="Screw 4 Status"() -> (w199:refnum<vi>)
            n92 = control-ref of="Screw 5 Status"() -> (w198:refnum<vi>)
            n93 = control-ref of="Screw 6 Status"() -> (w197:refnum<vi>)
            n94 = control-ref of="Final Result"() -> (w196:refnum<vi>)
            n95 = control-ref of="Final Result"() -> (w193:refnum<vi>)
            n96 = call "OP50 Indicators.vi"("error in (no error)"=w213, "Array"=w206, "OUTPUT INDICATOR"=w212) -> ("error out"=w205:errorcluster, "OUTPUT INDICATOR"=w204:T14)  [unwired: 7 in]
            n97 = Build Array(w202, w201, w200, w199, w198, w197, w196) -> (w203:refnum<vi>[])
            n98 = control-ref of="Loctite Status"() -> (w189:refnum<vi>)
            n99 = control-ref of="Final Result"() -> (w188:refnum<vi>)
            n100 = Build Array(w193) -> (w192:refnum<vi>[])
            n101 = call "OP60 Indicators.vi"("error in (no error)"=w205, "Array"=w203, "OUTPUT INDICATOR"=w204) -> ("error out"=w195:errorcluster, "OUTPUT INDICATOR"=w194:T14)  [unwired: 7 in]
            n102 = call "OP70 Indicators.vi"("error in (no error)"=w195, "Array"=w192, "OUTPUT INDICATOR"=w194) -> ("error out"=w191:errorcluster, "OUTPUT INDICATOR"=w190:T14)  [unwired: 7 in]
            n103 = control-ref of="Seat Status"() -> (w184:refnum<vi>)
            n104 = control-ref of="Final Result"() -> (w183:refnum<vi>)
            n105 = control-ref of="Final Result"() -> (w179:refnum<vi>)
            n106 = control-ref of="Camera Status"() -> (w171:refnum<vi>)
            n107 = Build Array(w189, w188) -> (w187:refnum<vi>[])
            n108 = call "OP80 Indicators.vi"("error in (no error)"=w191, "Array"=w187, "OUTPUT INDICATOR"=w190) -> ("error out"=w185:errorcluster, "OUTPUT INDICATOR"=w186:T14)  [unwired: 7 in]
            n109 = Build Array(w184, w183) -> (w182:refnum<vi>[])
            n110 = Build Array(w179, w171) -> (w178:refnum<vi>[])
            n111 = call "OP90 Indicators.vi"("error in (no error)"=w185, "Array"=w182, "OUTPUT INDICATOR"=w186) -> ("error out"=w181:errorcluster, "OUTPUT INDICATOR"=w180:T14)  [unwired: 7 in]
            n112 = call "OP100 Indicators.vi"("error in (no error)"=w181, "Array"=w178, "OUTPUT INDICATOR"=w180) -> ("error out"=w172:errorcluster, "OUTPUT INDICATOR"=w177:T14)  [unwired: 7 in]
            n113 = call "PADMINI_AUTO_BARCODE_STRING 110.vi"("Enum"=enum16{"Read", "Write"}."Read", "error in (no error)"=w172) -> ("Input 2"=w174:string[])  [unwired: 8 in, 1 out]
            n114 = Index Array(array=w174) -> (element=w175:string)  [unwired: 1 in]
            n115 = Bundle By Name(cluster=w177, "OP - 110.BARCODE"=w175) -> (w176:T14)
          }
          frame "SCAN1" {
            # "STATION OP 10"
            n116 = global read "Global 1.vi" "BARCODE RECIPE"() -> (w249:string)
            n117 = call "PADMINI_AUTO_BARCODE_STRING.vi"("Enum"=enum16{"Read", "Write"}."Read", "error in (no error)"=w258) -> ("error out"=w257:errorcluster, "Input 2"=w245:string[])  [unwired: 8 in]
            n118 = Index Array(array=w245) -> (element=w244:string)  [unwired: 1 in]
            n119 = call <vilib>:"Trim Whitespace.vi"("string"=w244) -> ("trimmed string"=w243:string)  [unwired: 1 in]
            n120 = Match Pattern(string=w243, regular expression=w249) -> (match substring=w252:string)  [unwired: 1 in, 3 out]
            n121 = String Length(string=w249) -> (length=w251:i32)
            n122 = String Length(string=w252) -> (length=w250:i32)
            n123 = Equal?(x=w251, y=w250) -> (x = y?=w256:bool)
            n124 = case shown="False" w255 {
              tunnel: w262 -> [w288 w306]
              tunnel: w257 -> [w287 w304]
              tunnel: w261 -> [w286 _]
              tunnel: [w285 w303] -> w247
              tunnel: [w284 w306] -> w260
              tunnel: w256 -> [_ _]
              tunnel: w243 -> [w283 _]
              tunnel: [w282 TRUE] -> w241
              frame False {
                n125 = Format Into String(format string="where BARCODE='%s'", w283) -> (resulting string=w279:string)  [unwired: 2 in, 1 out]
                n126 = call <vilib>:"DB Tools Select Data.vi"("condition"=w279, "error in (no error)"=w287, "columns"=string[] ["BARCODE", "OP10_FINAL_RESULT"], "table"=w286, "connection reference"=w288) -> ("error out"=w278:errorcluster, "data"=w277:variant[][], "connection reference out"=w284:T13)  [unwired: 1 in]
                n127 = call "PADMINI_varient_to_data.vi"("error in (no error)"=w278, "data"=w277) -> ("error out"=w275:errorcluster, "Array"=w271:string[][])  [unwired: 8 in]
                n128 = Index Array(array=w271, index (row)=0) -> (element=→"SCAN OP10":string[])  [unwired: 1 in]
                n129 = Index Array(array=w271, index (row)=0, index (col)=1 ("index (row)")) -> (element=w272:string)
                n130 = Empty Array?(array=w271) -> (empty?=w276:bool)
                n131 = case shown="False" w276 {
                  tunnel: w275 -> [w298 w300]
                  tunnel: [w297 w300] -> w285
                  tunnel: [FALSE TRUE] -> w282
                  tunnel: w272 -> [w292 _]
                  frame False {
                    w291 = "OK"  # y
                    w294 = i32[] [1, 0]  # I/P
                    w293 = i32[] [0, 1]  # I/P
                    # "OP10 CURRENT STATION OK-NG\nPART REPEAT"
                    n132 = Equal?(x=w292, y=w291) -> (x = y?=w290:bool)
                    n133 = Select(t=w294, s=w290, f=w293) -> (s? t:f=w289:i32[])
                    "OP10 STATUS" <- w289
                    n134 = call "PADMINI_AUTO_BARCODE_STATUS.vi"("Enum"=enum16{"Read", "Write"}."Write", "error in (no error)"=w298, "I/P"=w289) -> ("error out"=w297:errorcluster)  [unwired: 7 in, 1 out]
                  }
                  frame True {
                    # "OP10 NEW part"
                  }
                }
              }
              frame True {
                w302 = i32[] [0, 1]  # I/P
                n135 = call "PADMINI_AUTO_BARCODE_STATUS.vi"("Enum"=enum16{"Read", "Write"}."Write", "error in (no error)"=w304, "I/P"=w302) -> ("error out"=w303:errorcluster)  [unwired: 7 in, 1 out]
              }
            }
            n136 = flat-sequence {
              tunnel: [w268] -> w246
              tunnel: w247 -> [w268]
              frame #0 {
                # "UPDATE op 10 sCAN sTATUS"
                n137 = global write "DATA LOG.vi" "OP 10 Outputs"(TRUE) -> ()
              }
            }
            n138 = call <vilib>:"Clear Errors.vi"("error in (no error)"=w246) -> ("error out"=w240:errorcluster)  [unwired: 5 in, 1 out]
            n139 = case shown="True" w241 {
              tunnel: w242 -> [_ w266]
              tunnel: w240 -> [_ w264]
              frame False {
              }
              frame True {
                w265 = cluster{"CASE 2":T12} {"CASE 2"=enum."DATALOG1"}  # element
                n140 = Enqueue Element(queue=w266, element=w265, error in (no error)=w264) -> ()  [unwired: 1 in, 3 out]
              }
            }
          }
          frame "DATALOG1" {
            w321 = T15 2 items=["no dialog", "OK message", "continue or stop message", "OK message + warnings", "continue/stop + warnings"] ("type of dialog (OK msg:1)")
            # "cycle result status\nwhether it was ok or nok\nor abortted in between"
            # "Printed QR Code data string"
            # "datalog of OP 10"
            n141 = call "PADMINI_AUTO_BARCODE_STRING.vi"("Enum"=enum16{"Read", "Write"}."Read", "error in (no error)"=w307) -> ("Input 2"=w314:string[])  [unwired: 8 in, 1 out]
            n142 = call "PADMINI_AUTO_CYCLE VALUE 10.vi"("Enum"=enum16{"Read", "Write"}."Read", "error in (no error)"=w307) -> ("error out"=w310:errorcluster, "Input 2"=w309:sgl[])  [unwired: 8 in]
            n143 = Index Array(array=w309) -> (element=w308:sgl)  [unwired: 1 in]
            n144 = Index Array(array=w314) -> (element #1=w313:string, element #2=w312:string)  [unwired: 2 in]
            n145 = Number To Fractional String(number=w308, precision (6)=i16 2) -> (F-format string=w315:string)  [unwired: 2 in]
            n146 = call <vilib>:"Trim Whitespace.vi"("string"=w313) -> ("trimmed string"=w324:string)  [unwired: 1 in]
            n147 = case shown="False" w329 {
              tunnel: w330 -> [w354 w389]
              tunnel: w310 -> [w356 w388]
              tunnel: [w362 w387] -> w327
              tunnel: [w361 w386] -> w322
              tunnel: w328 -> [w351 _]
              tunnel: w324 -> [w348 _]
              tunnel: w312 -> [w358 w379]
              tunnel: w315 -> [w342 w378]
              frame False {
                w350 = string[] ["BARCODE", "SHIFT", "OP10_DATE", "OP10_LEAK_RATE_SCCM", "OP10_FINAL_RESULT"]
                # "ST1 RESULT"
                # "DO TRACEBILITY"
                n148 = local read "SHIFT"() -> (w360:string)
                n149 = Format Into String(format string="Where BARCODE='%s' ", w348) -> (resulting string=w343:string)  [unwired: 2 in, 1 out]
                n150 = call <vilib>:"DB Tools Select Data.vi"("condition"=w343, "error in (no error)"=w356, "columns"=w350, "table"=w351, "connection reference"=w354) -> ("error out"=w352:errorcluster, "data"=w355:variant[][], "connection reference out"=w353:T13)  [unwired: 1 in]
                n151 = call "PADMINI_SHIFT_DATE.vi"("SHIFT"=w360) -> ("date/time string"=w359:string)  [unwired: 10 in]
                n152 = Variant To Data(error in=w352, type=string[][] [], Variant=w355) -> (data=w346:string[][], error out=w344:errorcluster)
                n153 = Bundle("trimmed string"=w348, "SHIFT"=w360, "date/time string"=w359, w342, "Input 2"=w358) -> (w357:T16)  [unwired: 1 in]
                n154 = Empty Array?(array=w346) -> (empty?=w345:bool)
                n155 = case shown="False" w345 {
                  tunnel: w353 -> [w367 w377]
                  tunnel: w344 -> [w366 w376]
                  tunnel: [w370 w375] -> w362
                  tunnel: [w369 w374] -> w361
                  tunnel: w350 -> [w364 w373]
                  tunnel: w351 -> [w365 w372]
                  tunnel: w357 -> [w368 w371]
                  tunnel: w343 -> [w363 _]
                  frame False {
                    n156 = call <vilib>:"DB Tools Update Data.vi"("condition"=w363, "data"=w368, "error in (no error)"=w366, "columns"=w364, "table"=w365, "connection reference"=w367) -> ("error out"=w369:errorcluster, "connection reference out"=w370:T13)  [unwired: 4 in]
                  }
                  frame True {
                    n157 = call <vilib>:"DB Tools Insert Data.vi"("data"=w371, "error in (no error)"=w376, "columns"=w373, "table"=w372, "connection reference"=w377) -> ("error out"=w374:errorcluster, "connection reference out"=w375:T13)  [unwired: 5 in]
                  }
                }
              }
              frame True {
                # "Trac BYPASS"
                n158 = local read "SHIFT"() -> (w384:string)
                n159 = call "PADMINI_SHIFT_DATE.vi"("SHIFT"=w384) -> ("date/time string"=w383:string)  [unwired: 10 in]
                n160 = Bundle("SHIFT"=w384, "date/time string"=w383, "Input 2"=w379, w378) -> (w382:T17)  [unwired: 1 in]
                n161 = To Variant(anything=w382) -> (Variant=w381:variant)
                n162 = call <vilib>:"DB Tools Insert Data.vi"("data"=w381, "error in (no error)"=w388, "columns"=string[] ["DATE", "SHIFT", "OP10_LEAK_RAT", "OP10_FINAL_RST"], "table"="ST1_REPORT", "connection reference"=w389) -> ("error out"=w386:errorcluster, "connection reference out"=w387:T13)  [unwired: 5 in]
              }
            }
            n163 = call <vilib>:"Simple Error Handler.vi"("type of dialog (OK msg:1)"=w321, "error in (no error)"=w322) -> ("error out"=w320:errorcluster)  [unwired: 3 in, 4 out]
            n164 = call <vilib>:"Clear Errors.vi"("error in (no error)"=w320) -> ("error out"=w318:errorcluster)  [unwired: 5 in, 1 out]
            n165 = disable-structure shown="Enabled" {
              disable-tunnel: [w340 w341] -> w326
              disable-tunnel: w318 -> [w339 w341]
              frame Disabled {
                w334 = refnum<vi> refnum  # Boolean
                n166 = property on="OP - 10" class="Clust"(error in=w339) -> (error out=w333:errorcluster, "Controls[]"=w337:refnum<vi>[])  [unwired: 1 in, 1 out]
                n167 = Index Array(array=w337, index=2) -> (element=w335:refnum<vi>)
                n168 = To More Specific Class(target class=w334, reference=w335, error in=w333) -> (specific class reference=w338:refnum<vi>, error out=w332:errorcluster)
                n169 = call "PADMINI_BOOL_COLOR_CHANGE.vi"("error in (no error)"=w332, "Boolean in"=w338) -> ("error out"=w340:errorcluster)  [unwired: 9 in]
              }
              frame Enabled {
              }
            }
          }
          frame "SCAN2" {
            # "Barcode Status\n0-Ideal, 1-Ok, 2-Nok, 3-Prev Station Not Done,\n4-Prev Station Nok,\n5- Already Done"
            # "STATION OP 20"
            n170 = case shown="False" w396 {
              tunnel: w400 -> [w425 w431]
              tunnel: w399 -> [w418 w429]
              tunnel: w398 -> [w406 _]
              tunnel: [w420 w428] -> w395
              tunnel: [w419 w431] -> w397
              tunnel: [w407 "" ("trimmed string")] -> _
              frame False {
                # "ST2 RESULT"
                # "ST1 RESULT"
                # "2 FOR EMPTY BARCODE READ OR MISMATCH"
                n171 = call "PADMINI_AUTO_BARCODE_STRING2.vi"("Enum"=enum16{"Read", "Write"}."Read", "error in (no error)"=w418) -> ("error out"=w417:errorcluster, "Input 2"=w409:string[])  [unwired: 8 in]
                n172 = global read "Global 1.vi" "BARCODE RECIPE"() -> (w410:string)
                n173 = Index Array(array=w409) -> (element=w408:string)  [unwired: 1 in]
                n174 = call <vilib>:"Trim Whitespace.vi"("string"=w408) -> ("trimmed string"=w407:string)  [unwired: 1 in]
                n175 = Match Pattern(string=w407, regular expression=w410) -> (match substring=w411:string)  [unwired: 1 in, 3 out]
                n176 = String Length(string=w410) -> (length=w413:i32)
                n177 = String Length(string=w411) -> (length=w412:i32)
                n178 = Format Into String(format string="WHERE BARCODE  ='%s'", w407) -> (resulting string=w414:string)  [unwired: 2 in, 1 out]
                n179 = Equal?(x=w413, y=w412) -> ()  [unwired: 1 out]
                n180 = call <vilib>:"DB Tools Select Data.vi"("condition"=w414, "error in (no error)"=w417, "columns"=string[] ["BARCODE", "OP10_FINAL_RESULT", "OP20_FINAL_RESULT"], "table"=w406, "connection reference"=w425) -> ("error out"=w423:errorcluster, "data"=w422:variant[][], "connection reference out"=w419:T13)  [unwired: 1 in]
                n181 = call "PADMINI_varient_to_data.vi"("error in (no error)"=w423, "data"=w422) -> ("error out"=w421:errorcluster, "Array"=w403:string[][])  [unwired: 8 in]
                n182 = Index Array(array=w403, index (row)=0 ("disabled index (col)")) -> (element=→"SCAN OP20":string[])  [unwired: 1 in]
                n183 = call "RESPONSE_LOGIC.vi"("Array"=w403) -> ("Not Found"=w401:i32[])  [unwired: 10 in]
                "OP20 STATUS" <- w401
                n184 = call "PADMINI_AUTO_BARCODE_STATUS 20.vi"("Enum"=enum16{"Read", "Write"}."Write", "error in (no error)"=w421, "I/P"=w401) -> ("error out"=w420:errorcluster)  [unwired: 7 in, 1 out]
              }
              frame True {
                w426 = i32[] [0, 0, 0, 0, 0]  # I/P
                n185 = call "PADMINI_AUTO_BARCODE_STATUS 20.vi"("Enum"=enum16{"Read", "Write"}."Write", "error in (no error)"=w429, "I/P"=w426) -> ("error out"=w428:errorcluster)  [unwired: 7 in, 1 out]
              }
            }
            n186 = flat-sequence {
              tunnel: [w433] -> w394
              tunnel: w395 -> [w433]
              frame #0 {
                # "UPDATE op 20 SCAN sTATUS"
                n187 = global write "DATA LOG.vi" "OP 20 Outputs"(TRUE) -> ()
              }
            }
          }
          frame "DATALOG2" {
            (unwired) string[] ["OP20_DATE", "OP20_LOWER_BEARING_DIS", "OP20_LOWER_BEARING_LOAD", "OP20_UPPER_BEARING_DIS", "OP20_UPPER_BEARING_LOAD", "OP20_LOWER_BEARING_RST", "OP20_BOTTOM_CAMERA_STATUS", "OP20_UPPER_SIM_STATUS", "OP20_UPPER_BERAING_RST", "OP20_UPPER_CAMERA_STATUS", "OP20_FINAL_RST"]
            w447 = T15 2 items=["no dialog", "OK message", "continue or stop message", "OK message + warnings", "continue/stop + warnings"] ("type of dialog (OK msg:1)")
            # "Printed QR Code data string"
            # "datalog of OP 20"
            n188 = call "PADMINI_AUTO_BARCODE_STRING2.vi"("Enum"=enum16{"Read", "Write"}."Read", "error in (no error)"=w440) -> ("error out"=w442:errorcluster, "Input 2"=w436:string[])  [unwired: 8 in]
            n189 = call "PADMINI_AUTO_CYCLE VALUE 20.vi"("Enum"=enum16{"Read", "Write"}."Read", "error in (no error)"=w440) -> ("Input 2"=w438:sgl[])  [unwired: 8 in, 1 out]
            n190 = Number To Fractional String(number=w438, precision (6)=i16 2) -> (F-format string=w437:string[])  [unwired: 2 in]
            n191 = case shown="False" w452 {
              tunnel: w453 -> [w477 w503]
              tunnel: w442 -> [w478 w502]
              tunnel: [w481 w501] -> w450
              tunnel: [w480 w500] -> w448
              tunnel: w451 -> [w476 _]
              tunnel: w437 -> [w473 w485]
              tunnel: w436 -> [w467 w486]
              frame False {
                # "ST2 RESULT"
                # "DO TRACEBILITY"
                n192 = Index Array(array=w467) -> (element #1=w468:string, element #2=w463:string, element #3=w462:string, element #4=w461:string, element #5=w460:string, element #6=w459:string, element #7=w458:string)  [unwired: 7 in]
                n193 = local read "SHIFT"() -> (w479:string)
                n194 = Index Array(array=w473) -> (element #1=w472:string, element #2=w471:string, element #3=w465:string, element #4=w464:string)  [unwired: 4 in]
                n195 = call <vilib>:"Trim Whitespace.vi"("string"=w468) -> ("trimmed string"=w469:string)  [unwired: 1 in]
                n196 = call "PADMINI_SHIFT_DATE.vi"("SHIFT"=w479) -> ("date/time string"=w466:string)  [unwired: 10 in]
                n197 = Format Into String(format string="Where BARCODE='%s' ", w469) -> (resulting string=w474:string)  [unwired: 2 in, 1 out]
                n198 = Bundle("date/time string"=w466, "Input 2"=w472, "Input 2"=w471, "Input 2"=w465, "Input 2"=w464, "Input 2"=w463, "Input 2"=w462, "Input 2"=w461, "Input 2"=w460, "Input 2"=w459, "Input 2"=w458) -> (w470:T18)  [unwired: 1 in]
                n199 = call <vilib>:"DB Tools Update Data.vi"("condition"=w474, "data"=w470, "error in (no error)"=w478, "columns"=string[] ["OP20_DATE", "OP20_BOTTOM_DISPLACE_mm", "OP20_BOTTOM_LOAD_kg", "OP20_TOP_DISPLACE_mm", "OP20_TOP_LOAD_kg", "OP20_BOTTOM_RESULT", "OP20_BOTTOM_CAMERA_STATUS", "OP20_TOP_SIM_STATUS", "OP20_TOP_RESULT", "OP20_TOP_CAMERA_STATUS", "OP20_FINAL_RESULT"], "table"=w476, "connection reference"=w477) -> ("error out"=w480:errorcluster, "connection reference out"=w481:T13)  [unwired: 4 in]
              }
              frame True {
                n200 = local read "SHIFT"() -> (w483:string)
                n201 = Index Array(array=w486) -> (element #2=w492:string, element #3=w491:string, element #4=w490:string, element #5=w489:string, element #6=w488:string, element #7=w482:string)  [unwired: 7 in, 1 out]
                n202 = call "PADMINI_SHIFT_DATE.vi"("SHIFT"=w483) -> ("date/time string"=w484:string)  [unwired: 10 in]
                n203 = Index Array(array=w485) -> (element #1=w496:string, element #2=w495:string, element #3=w494:string, element #4=w493:string)  [unwired: 4 in]
                n204 = Bundle("date/time string"=w484, "SHIFT"=w483, "Input 2"=w496, "Input 2"=w495, "Input 2"=w492, "Input 2"=w491, "Input 2"=w494, "Input 2"=w493, "Input 2"=w490, "Input 2"=w489, "Input 2"=w488, "Input 2"=w482) -> (w487:T19)  [unwired: 1 in]
                n205 = To Variant(anything=w487) -> (Variant=w498:variant)
                n206 = call <vilib>:"DB Tools Insert Data.vi"("data"=w498, "error in (no error)"=w502, "columns"=string[] ["DATE", "SHIFT", "ST2_LOWER_BEARING_DIS", "ST2_LOWER_BEARING_LOAD", "ST2_BOTTOM_CAMERA_STATUS", "ST2_LOWER_BEARING_RST", "ST2_UPPER_BEARING_DIS", "ST2_UPPER_BEARING_LOAD", "ST2_UPPER_SIM_STATUS", "ST2_UPPER_CAMERA_STATUS", "ST2_UPPER_BERAING_RST", "ST2_FINAL_RST"], "table"="ST2_REPORT", "connection reference"=w503) -> ("error out"=w500:errorcluster, "connection reference out"=w501:T13)  [unwired: 5 in]
              }
            }
            n207 = call <vilib>:"Simple Error Handler.vi"("type of dialog (OK msg:1)"=w447, "error in (no error)"=w448) -> ("error out"=w446:errorcluster)  [unwired: 3 in, 4 out]
            n208 = call <vilib>:"Clear Errors.vi"("error in (no error)"=w446) -> ("error out"=w444:errorcluster)  [unwired: 5 in, 1 out]
            n209 = flat-sequence {
              tunnel: [w456] -> w435
              tunnel: w444 -> [w456]
              frame #0 {
                # "UPDATE op 20 save"
                n210 = global write "DATA LOG.vi" "OP 20 reset"(TRUE) -> ()
              }
            }
          }
          frame "SCAN3" {
            # "STATION OP 30"
            n211 = case shown="False" w510 {
              tunnel: w514 -> [w540 w546]
              tunnel: w513 -> [w533 w544]
              tunnel: w512 -> [w520 _]
              tunnel: [w535 w543] -> w509
              tunnel: [w534 w546] -> w511
              tunnel: [w521 "" ("trimmed string")] -> _
              frame False {
                n212 = call "PADMINI_AUTO_BARCODE_STRING 30.vi"("Enum"=enum16{"Read", "Write"}."Read", "error in (no error)"=w533) -> ("error out"=w532:errorcluster, "Input 2"=w523:string[])  [unwired: 8 in]
                n213 = global read "Global 1.vi" "BARCODE RECIPE"() -> (w524:string)
                n214 = Index Array(array=w523) -> (element=w522:string)  [unwired: 1 in]
                n215 = call <vilib>:"Trim Whitespace.vi"("string"=w522) -> ("trimmed string"=w521:string)  [unwired: 1 in]
                n216 = Match Pattern(string=w521, regular expression=w524) -> (match substring=w525:string)  [unwired: 1 in, 3 out]
                n217 = String Length(string=w524) -> (length=w527:i32)
                n218 = String Length(string=w525) -> (length=w526:i32)
                n219 = Equal?(x=w521, y="") -> ()  [unwired: 1 out]
                n220 = Format Into String(format string="WHERE BARCODE  ='%s'", w521) -> (resulting string=w529:string)  [unwired: 2 in, 1 out]
                n221 = Equal?(x=w527, y=w526) -> ()  [unwired: 1 out]
                n222 = call <vilib>:"DB Tools Select Data.vi"("condition"=w529, "error in (no error)"=w532, "columns"=string[] ["BARCODE", "OP20_FINAL_RESULT", "OP30_FINAL_RESULT"], "table"=w520, "connection reference"=w540) -> ("error out"=w538:errorcluster, "data"=w537:variant[][], "connection reference out"=w534:T13)  [unwired: 1 in]
                n223 = call "PADMINI_varient_to_data.vi"("error in (no error)"=w538, "data"=w537) -> ("error out"=w536:errorcluster, "Array"=w517:string[][])  [unwired: 8 in]
                n224 = Index Array(array=w517, index (row)=0 ("disabled index (col)")) -> (element=→"SCAN OP30":string[])  [unwired: 1 in]
                n225 = call "RESPONSE_LOGIC.vi"("Array"=w517) -> ("Not Found"=w515:i32[])  [unwired: 10 in]
                "OP30 STATUS" <- w515
                n226 = call "PADMINI_AUTO_BARCODE_STATUS 30.vi"("Enum"=enum16{"Read", "Write"}."Write", "error in (no error)"=w536, "I/P"=w515) -> ("error out"=w535:errorcluster)  [unwired: 7 in, 1 out]
              }
              frame True {
                w541 = i32[] [0, 0, 0, 0, 0]  # I/P
                n227 = call "PADMINI_AUTO_BARCODE_STATUS 30.vi"("Enum"=enum16{"Read", "Write"}."Write", "error in (no error)"=w544, "I/P"=w541) -> ("error out"=w543:errorcluster)  [unwired: 7 in, 1 out]
              }
            }
            n228 = flat-sequence {
              tunnel: [w548] -> w508
              tunnel: w509 -> [w548]
              frame #0 {
                # "UPDATE op 30 SCAN sTATUS"
                n229 = global write "DATA LOG.vi" "OP 30 Outputs"(TRUE) -> ()
              }
            }
          }
          frame "DATALOG3" {
            (unwired) string[] ["OP30_DATE", "OP30_DISPLACEMENT", "OP30_SHAFT_PRESS_LOAD", "OP30_SHAFT_STATUS", "OP30_FINAL_RST"]
            w562 = T15 2 items=["no dialog", "OK message", "continue or stop message", "OK message + warnings", "continue/stop + warnings"] ("type of dialog (OK msg:1)")
            # "Printed QR Code data string"
            # "datalog of OP 30"
            n230 = call "PADMINI_AUTO_BARCODE_STRING 30.vi"("Enum"=enum16{"Read", "Write"}."Read", "error in (no error)"=w554) -> ("error out"=w556:errorcluster, "Input 2"=w550:string[])  [unwired: 8 in]
            n231 = call "PADMINI_AUTO_CYCLE VALUE 30.vi"("Enum"=enum16{"Read", "Write"}."Read", "error in (no error)"=w554) -> ("Input 2"=w552:sgl[])  [unwired: 8 in, 1 out]
            n232 = Number To Fractional String(number=w552, precision (6)=i16 2) -> (F-format string=w551:string[])  [unwired: 2 in]
            n233 = case shown="False" w567 {
              tunnel: w568 -> [w586 w606]
              tunnel: w556 -> [w587 w605]
              tunnel: [w590 w604] -> w565
              tunnel: [w589 w603] -> w563
              tunnel: w566 -> [w585 _]
              tunnel: w551 -> [w582 w591]
              tunnel: w550 -> [w576 w592]
              frame False {
                # "DO TRACEBILITY"
                n234 = Index Array(array=w576) -> (element #1=w577:string, element #2=w575:string, element #3=w574:string)  [unwired: 3 in]
                n235 = local read "SHIFT"() -> (w588:string)
                n236 = Index Array(array=w582) -> (element #1=w581:string, element #2=w580:string)  [unwired: 2 in]
                n237 = call <vilib>:"Trim Whitespace.vi"("string"=w577) -> ("trimmed string"=w578:string)  [unwired: 1 in]
                n238 = call "PADMINI_SHIFT_DATE.vi"("SHIFT"=w588) -> ("date/time string"=w573:string)  [unwired: 10 in]
                n239 = Format Into String(format string="Where BARCODE='%s' ", w578) -> (resulting string=w583:string)  [unwired: 2 in, 1 out]
                n240 = Bundle("date/time string"=w573, "Input 2"=w581, "Input 2"=w580, "Input 2"=w575, "Input 2"=w574) -> (w579:T20)  [unwired: 1 in]
                n241 = call <vilib>:"DB Tools Update Data.vi"("condition"=w583, "data"=w579, "error in (no error)"=w587, "columns"=string[] ["OP30_DATE", "OP30_DISPLACEMENT_mm", "OP30_SHAFT_PRESS_LOAD_kg", "OP30_SHAFT_STATUS", "OP30_FINAL_RESULT"], "table"=w585, "connection reference"=w586) -> ("error out"=w589:errorcluster, "connection reference out"=w590:T13)  [unwired: 4 in]
              }
              frame True {
                # "TRAC BYPASS"
                n242 = local read "SHIFT"() -> (w593:string)
                n243 = call "PADMINI_SHIFT_DATE.vi"("SHIFT"=w593) -> ("date/time string"=w594:string)  [unwired: 10 in]
                n244 = Index Array(array=w592) -> (element #2=w598:string, element #3=w597:string)  [unwired: 3 in, 1 out]
                n245 = Index Array(array=w591) -> (element #1=w600:string, element #2=w599:string)  [unwired: 2 in]
                n246 = Bundle("date/time string"=w594, "SHIFT"=w593, "Input 2"=w600, "Input 2"=w599, "Input 2"=w598, "Input 2"=w597) -> (w595:T21)  [unwired: 1 in]
                n247 = To Variant(anything=w595) -> (Variant=w596:variant)
                n248 = call <vilib>:"DB Tools Insert Data.vi"("data"=w596, "error in (no error)"=w605, "columns"=string[] ["DATE", "SHIFT", "ST3_DISPLACEMENT", "ST3_LOAD", "ST3_MIDDLE_GEAR_SHAFT_STATUS", "ST3_FINAL_RST"], "table"="ST3_REPORT", "connection reference"=w606) -> ("error out"=w603:errorcluster, "connection reference out"=w604:T13)  [unwired: 5 in]
              }
            }
            n249 = call <vilib>:"Simple Error Handler.vi"("type of dialog (OK msg:1)"=w562, "error in (no error)"=w563) -> ("error out"=w561:errorcluster)  [unwired: 3 in, 4 out]
            n250 = call <vilib>:"Clear Errors.vi"("error in (no error)"=w561) -> ("error out"=w559:errorcluster)  [unwired: 5 in, 1 out]
            n251 = flat-sequence {
              tunnel: [w571] -> w549
              tunnel: w559 -> [w571]
              frame #0 {
                # "UPDATE op 20 save"
                n252 = global write "DATA LOG.vi" "OP 30 reset"(TRUE) -> ()
              }
            }
          }
          frame "SCAN4" {
            # "STATION OP 40"
            n253 = case shown="False" w613 {
              tunnel: w617 -> [w638 w644]
              tunnel: w616 -> [w631 w643]
              tunnel: w615 -> [w623 _]
              tunnel: [w633 w642] -> w612
              tunnel: [w632 w644] -> w614
              tunnel: [w624 "" ("trimmed string")] -> _
              frame False {
                n254 = call "PADMINI_AUTO_BARCODE_STRING 40.vi"("Enum"=enum16{"Read", "Write"}."Read", "error in (no error)"=w631) -> ("error out"=w630:errorcluster, "Input 2"=w626:string[])  [unwired: 8 in]
                n255 = Index Array(array=w626) -> (element=w625:string)  [unwired: 1 in]
                n256 = call <vilib>:"Trim Whitespace.vi"("string"=w625) -> ("trimmed string"=w624:string)  [unwired: 1 in]
                n257 = Format Into String(format string="WHERE BARCODE  ='%s'", w624) -> (resulting string=w627:string)  [unwired: 2 in, 1 out]
                n258 = call <vilib>:"DB Tools Select Data.vi"("condition"=w627, "error in (no error)"=w630, "columns"=string[] ["BARCODE", "OP30_FINAL_RESULT", "OP40_FINAL_RESULT"], "table"=w623, "connection reference"=w638) -> ("error out"=w636:errorcluster, "data"=w635:variant[][], "connection reference out"=w632:T13)  [unwired: 1 in]
                n259 = call "PADMINI_varient_to_data.vi"("error in (no error)"=w636, "data"=w635) -> ("error out"=w634:errorcluster, "Array"=w620:string[][])  [unwired: 8 in]
                n260 = call "RESPONSE_LOGIC.vi"("Array"=w620) -> ("Not Found"=w618:i32[])  [unwired: 10 in]
                "OP40 STATUS" <- w618
                n261 = Index Array(array=w620, index (row)=0 ("disabled index (col)")) -> (element=→"SCAN OP40":string[])  [unwired: 1 in]
                n262 = call "PADMINI_AUTO_BARCODE_STATUS 40.vi"("Enum"=enum16{"Read", "Write"}."Write", "error in (no error)"=w634, "I/P"=w618) -> ("error out"=w633:errorcluster)  [unwired: 7 in, 1 out]
              }
              frame True {
                w639 = i32[] [0, 0, 0, 0, 0]  # I/P
                n263 = call "PADMINI_AUTO_BARCODE_STATUS 40.vi"("Enum"=enum16{"Read", "Write"}."Write", "error in (no error)"=w643, "I/P"=w639) -> ("error out"=w642:errorcluster)  [unwired: 7 in, 1 out]
              }
            }
            n264 = flat-sequence {
              tunnel: [w646] -> w611
              tunnel: w612 -> [w646]
              frame #0 {
                # "UPDATE op 40 SCAN sTATUS"
                n265 = global write "DATA LOG.vi" "OP 40 Outputs"(TRUE) -> ()
              }
            }
          }
          frame "DATALOG4" {
            w660 = T15 2 items=["no dialog", "OK message", "continue or stop message", "OK message + warnings", "continue/stop + warnings"] ("type of dialog (OK msg:1)")
            # "datalog of OP 40"
            n266 = call "PADMINI_AUTO_BARCODE_STRING 40.vi"("Enum"=enum16{"Read", "Write"}."Read", "error in (no error)"=w652) -> ("error out"=w654:errorcluster, "Input 2"=w648:string[])  [unwired: 8 in]
            n267 = call "PADMINI_AUTO_CYCLE VALUE 40.vi"("Enum"=enum16{"Read", "Write"}."Read", "error in (no error)"=w652) -> ("Input 2"=w650:sgl[])  [unwired: 8 in, 1 out]
            n268 = Number To Fractional String(number=w650, precision (6)=i16 2) -> (F-format string=w649:string[])  [unwired: 2 in]
            n269 = case shown="False" w665 {
              tunnel: w666 -> [w688 w712]
              tunnel: w654 -> [w689 w711]
              tunnel: [w692 w710] -> w663
              tunnel: [w691 w709] -> w661
              tunnel: w664 -> [w687 _]
              tunnel: w649 -> [w683 w694]
              tunnel: w648 -> [w678 w693]
              frame False {
                # "DO TRACEBILITY"
                n270 = Index Array(array=w678) -> (element #1=w679:string, element #2=w674:string, element #3=w673:string, element #4=w671:string, element #5=w670:string)  [unwired: 5 in]
                n271 = local read "SHIFT"() -> (w690:string)
                n272 = Index Array(array=w683) -> (element #1=w682:string, element #2=w677:string, element #3=w676:string, element #4=w675:string)  [unwired: 4 in]
                n273 = call <vilib>:"Trim Whitespace.vi"("string"=w679) -> ("trimmed string"=w680:string)  [unwired: 1 in]
                n274 = call "PADMINI_SHIFT_DATE.vi"("SHIFT"=w690) -> ("date/time string"=w672:string)  [unwired: 10 in]
                n275 = Format Into String(format string="Where BARCODE='%s' ", w680) -> (resulting string=w685:string)  [unwired: 2 in, 1 out]
                n276 = Bundle("date/time string"=w672, "Input 2"=w682, "Input 2"=w674, "Input 2"=w677, "Input 2"=w673, "Input 2"=w676, "Input 2"=w675, "Input 2"=w671, "Input 2"=w670) -> (w681:T22)  [unwired: 1 in]
                n277 = call <vilib>:"DB Tools Update Data.vi"("condition"=w685, "data"=w681, "error in (no error)"=w689, "columns"=string[] ["OP40_DATE", "OP40_RH_SCREW_Nm", "OP40_RH_STATUS", "OP40_LH_SCREW_Nm", "OP40_LH_STATUS", "OP40_DISPLACEMENT_mm", "OP40_STACK_LOAD_kg", "OP40_TOP_BEARING_CAMERA_STAUS", "OP40_FINAL_RESULT"], "table"=w687, "connection reference"=w688) -> ("error out"=w691:errorcluster, "connection reference out"=w692:T13)  [unwired: 4 in]
              }
              frame True {
                # "TRAC BYPASS"
                n278 = local read "SHIFT"() -> (w695:string)
                n279 = Index Array(array=w693) -> (element #2=w703:string, element #3=w702:string, element #4=w701:string, element #5=w700:string)  [unwired: 5 in, 1 out]
                n280 = call "PADMINI_SHIFT_DATE.vi"("SHIFT"=w695) -> ("date/time string"=w696:string)  [unwired: 10 in]
                n281 = Index Array(array=w694) -> (element #1=w697:string, element #2=w706:string, element #3=w705:string, element #4=w704:string)  [unwired: 4 in]
                n282 = Bundle("date/time string"=w696, "SHIFT"=w695, "Input 2"=w697, "Input 2"=w703, "Input 2"=w706, "Input 2"=w702, "Input 2"=w705, "Input 2"=w704, "Input 2"=w700, "Input 2"=w701) -> (w699:T23)  [unwired: 1 in]
                n283 = To Variant(anything=w699) -> (Variant=w698:variant)
                n284 = call <vilib>:"DB Tools Insert Data.vi"("data"=w698, "error in (no error)"=w711, "columns"=string[] ["DATE", "SHIFT", "ST4_SCREW1_DATA", "ST4_SCREW1_STATUS", "ST4_SCREW2_DATA", "ST4_SCREW2_STATUS", "ST4_DISPLACEMENT", "ST4_LOAD", "ST4_TOP_BEARING_CAMERA_STAUS", "ST4_FINAL_RST"], "table"="ST4_REPORT", "connection reference"=w712) -> ("error out"=w709:errorcluster, "connection reference out"=w710:T13)  [unwired: 5 in]
              }
            }
            n285 = call <vilib>:"Simple Error Handler.vi"("type of dialog (OK msg:1)"=w660, "error in (no error)"=w661) -> ("error out"=w659:errorcluster)  [unwired: 3 in, 4 out]
            n286 = call <vilib>:"Clear Errors.vi"("error in (no error)"=w659) -> ("error out"=w657:errorcluster)  [unwired: 5 in, 1 out]
            n287 = flat-sequence {
              tunnel: [w669] -> w647
              tunnel: w657 -> [w669]
              frame #0 {
                # "UPDATE op 20 save"
                n288 = global write "DATA LOG.vi" "OP 40 reset"(TRUE) -> ()
              }
            }
          }
          frame "SCAN5" {
            # "STATION OP 50"
            n289 = case shown="False" w719 {
              tunnel: w723 -> [w744 w750]
              tunnel: w722 -> [w737 w749]
              tunnel: w721 -> [w729 _]
              tunnel: [w739 w748] -> w718
              tunnel: [w738 w750] -> w720
              tunnel: [w730 "" ("trimmed string")] -> _
              frame False {
                n290 = call "PADMINI_AUTO_BARCODE_STRING 50.vi"("Enum"=enum16{"Read", "Write"}."Read", "error in (no error)"=w737) -> ("error out"=w736:errorcluster, "Input 2"=w732:string[])  [unwired: 8 in]
                n291 = Index Array(array=w732) -> (element=w731:string)  [unwired: 1 in]
                n292 = call <vilib>:"Trim Whitespace.vi"("string"=w731) -> ("trimmed string"=w730:string)  [unwired: 1 in]
                n293 = Format Into String(format string="WHERE BARCODE  ='%s'", w730) -> (resulting string=w733:string)  [unwired: 2 in, 1 out]
                n294 = call <vilib>:"DB Tools Select Data.vi"("condition"=w733, "error in (no error)"=w736, "columns"=string[] ["BARCODE", "OP40_FINAL_RESULT", "OP50_FINAL_RESULT"], "table"=w729, "connection reference"=w744) -> ("error out"=w742:errorcluster, "data"=w741:variant[][], "connection reference out"=w738:T13)  [unwired: 1 in]
                n295 = call "PADMINI_varient_to_data.vi"("error in (no error)"=w742, "data"=w741) -> ("error out"=w740:errorcluster, "Array"=w726:string[][])  [unwired: 8 in]
                n296 = Index Array(array=w726, index (row)=0 ("disabled index (col)")) -> (element=→"SCAN OP50":string[])  [unwired: 1 in]
                n297 = call "RESPONSE_LOGIC.vi"("Array"=w726) -> ("Not Found"=w725:i32[])  [unwired: 10 in]
                "OP50 STATUS" <- w725
                n298 = call "PADMINI_AUTO_BARCODE_STATUS 50.vi"("Enum"=enum16{"Read", "Write"}."Write", "error in (no error)"=w740, "I/P"=w725) -> ("error out"=w739:errorcluster)  [unwired: 7 in, 1 out]
              }
              frame True {
                w745 = i32[] [0, 0, 0, 0, 0]  # I/P
                n299 = call "PADMINI_AUTO_BARCODE_STATUS 50.vi"("Enum"=enum16{"Read", "Write"}."Write", "error in (no error)"=w749, "I/P"=w745) -> ("error out"=w748:errorcluster)  [unwired: 7 in, 1 out]
              }
            }
            n300 = flat-sequence {
              tunnel: [w752] -> w717
              tunnel: w718 -> [w752]
              frame #0 {
                # "UPDATE op 50 SCAN sTATUS"
                n301 = global write "DATA LOG.vi" "OP 50 Outputs"(TRUE) -> ()
              }
            }
          }
          frame "DATALOG5" {
            (unwired) string[] ["OP50_DATE", "OP50_NUT_TORQUE_Nm", "OP50_NUT_STATUS", "OP50_LH_MOTOR_SCREW_Nm", "OP50_LH_STATUS", "OP50_RH_MOTOR_SCREW_Nm", "OP50_RH_STATUS", "OP50_CAMERA_STATUS", "OP50_FINAL_RESULT"]
            w766 = T15 2 items=["no dialog", "OK message", "continue or stop message", "OK message + warnings", "continue/stop + warnings"] ("type of dialog (OK msg:1)")
            # "datalog of OP 50"
            n302 = call "PADMINI_AUTO_BARCODE_STRING 50.vi"("Enum"=enum16{"Read", "Write"}."Read", "error in (no error)"=w759) -> ("error out"=w761:errorcluster, "Input 2"=w755:string[])  [unwired: 8 in]
            n303 = call "PADMINI_AUTO_CYCLE VALUE 50.vi"("Enum"=enum16{"Read", "Write"}."Read", "error in (no error)"=w759) -> ("Input 2"=w757:sgl[])  [unwired: 8 in, 1 out]
            n304 = Number To Fractional String(number=w757, precision (6)=i16 2) -> (F-format string=w756:string[])  [unwired: 2 in]
            n305 = case shown="False" w771 {
              tunnel: w772 -> [w794 w816]
              tunnel: w761 -> [w795 w815]
              tunnel: [w798 w814] -> w769
              tunnel: [w797 w813] -> w767
              tunnel: w770 -> [w793 _]
              tunnel: w756 -> [w790 w800]
              tunnel: w755 -> [w786 w799]
              frame False {
                # "DO TRACEBILITY"
                n306 = Index Array(array=w786) -> (element #1=w787:string, element #2=w782:string, element #3=w780:string, element #4=w778:string, element #5=w777:string, element #6=w776:string)  [unwired: 6 in]
                n307 = local read "SHIFT"() -> (w796:string)
                n308 = Index Array(array=w790) -> (element #1=w783:string, element #2=w781:string, element #3=w779:string)  [unwired: 3 in]
                n309 = call <vilib>:"Trim Whitespace.vi"("string"=w787) -> ("trimmed string"=w788:string)  [unwired: 1 in]
                n310 = call "PADMINI_SHIFT_DATE.vi"("SHIFT"=w796) -> ("date/time string"=w785:string)  [unwired: 10 in]
                n311 = Format Into String(format string="Where BARCODE='%s' ", w788) -> (resulting string=w791:string)  [unwired: 2 in, 1 out]
                n312 = Bundle("date/time string"=w785, "Input 2"=w783, "Input 2"=w782, "Input 2"=w781, "Input 2"=w780, "Input 2"=w779, "Input 2"=w778, "Input 2"=w777, "Input 2"=w776) -> (w789:T22)  [unwired: 1 in]
                n313 = call <vilib>:"DB Tools Update Data.vi"("condition"=w791, "data"=w789, "error in (no error)"=w795, "columns"=string[] ["OP50_DATE", "OP50_NUT_TORQUE_Nm", "OP50_NUT_STATUS", "OP50_RH_MOTOR_SCREW_Nm", "OP50_RH_STATUS", "OP50_LH_MOTOR_SCREW_Nm", "OP50_LH_STATUS", "OP50_CAMERA_STATUS", "OP50_FINAL_RESULT"], "table"=w793, "connection reference"=w794) -> ("error out"=w797:errorcluster, "connection reference out"=w798:T13)  [unwired: 4 in]
              }
              frame True {
                # "TRAC BYPASS"
                n314 = local read "SHIFT"() -> (w801:string)
                n315 = Index Array(array=w799) -> (element #2=w805:string, element #3=w804:string, element #4=w809:string)  [unwired: 4 in, 1 out]
                n316 = Index Array(array=w800) -> (element #1=w808:string, element #2=w807:string, element #3=w806:string)  [unwired: 3 in]
                n317 = call "PADMINI_SHIFT_DATE.vi"("SHIFT"=w801) -> ("date/time string"=w802:string)  [unwired: 10 in]
                n318 = Bundle("date/time string"=w802, "SHIFT"=w801, "Input 2"=w808, "Input 2"=w805, "Input 2"=w807, "Input 2"=w804, "Input 2"=w806, "Input 2"=w809) -> (w803:T24)  [unwired: 1 in]
                n319 = To Variant(anything=w803) -> (Variant=w812:variant)
                n320 = call <vilib>:"DB Tools Insert Data.vi"("data"=w812, "error in (no error)"=w815, "columns"=string[] ["DATE", "SHIFT", "ST5_SCREW1_DATA", "ST5_SCREW1_STATUS", "ST5_SCREW2_DATA", "ST5_SCREW2_STATUS", "ST5_SCREW3_DATA", "ST5_FINAL_RST"], "table"="ST5_REPORT", "connection reference"=w816) -> ("error out"=w813:errorcluster, "connection reference out"=w814:T13)  [unwired: 5 in]
              }
            }
            n321 = call <vilib>:"Simple Error Handler.vi"("type of dialog (OK msg:1)"=w766, "error in (no error)"=w767) -> ("error out"=w765:errorcluster)  [unwired: 3 in, 4 out]
            n322 = call <vilib>:"Clear Errors.vi"("error in (no error)"=w765) -> ("error out"=w763:errorcluster)  [unwired: 5 in, 1 out]
            n323 = flat-sequence {
              tunnel: [w775] -> w754
              tunnel: w763 -> [w775]
              frame #0 {
                # "UPDATE op 20 save"
                n324 = global write "DATA LOG.vi" "OP 50 reset"(TRUE) -> ()
              }
            }
          }
          frame "SCAN6" {
            # "STATION OP 60"
            n325 = case shown="False" w823 {
              tunnel: w827 -> [w848 w854]
              tunnel: w826 -> [w841 w853]
              tunnel: w825 -> [_ _]
              tunnel: [w843 w852] -> w822
              tunnel: [w842 w854] -> w824
              tunnel: [w833 "" ("trimmed string")] -> _
              frame False {
                n326 = call "PADMINI_AUTO_BARCODE_STRING 60.vi"("Enum"=enum16{"Read", "Write"}."Read", "error in (no error)"=w841) -> ("error out"=w840:errorcluster, "Input 2"=w835:string[])  [unwired: 8 in]
                n327 = Index Array(array=w835) -> (element=w834:string)  [unwired: 1 in]
                n328 = call <vilib>:"Trim Whitespace.vi"("string"=w834) -> ("trimmed string"=w833:string)  [unwired: 1 in]
                n329 = Format Into String(format string="WHERE BARCODE  ='%s'", w833) -> (resulting string=w836:string)  [unwired: 2 in, 1 out]
                n330 = call <vilib>:"DB Tools Select Data.vi"("condition"=w836, "error in (no error)"=w840, "columns"=string[] ["BARCODE", "OP50_FINAL_RESULT", "OP60_FINAL_RESULT"], "table"="REPORT", "connection reference"=w848) -> ("error out"=w846:errorcluster, "data"=w845:variant[][], "connection reference out"=w842:T13)  [unwired: 1 in]
                n331 = call "PADMINI_varient_to_data.vi"("error in (no error)"=w846, "data"=w845) -> ("error out"=w844:errorcluster, "Array"=w830:string[][])  [unwired: 8 in]
                n332 = Index Array(array=w830, index (row)=0 ("disabled index (col)")) -> (element=→"SCAN OP60":string[])  [unwired: 1 in]
                n333 = call "RESPONSE_LOGIC.vi"("Array"=w830) -> ("Not Found"=w828:i32[])  [unwired: 10 in]
                "OP60 STATUS" <- w828
                n334 = call "PADMINI_AUTO_BARCODE_STATUS 60.vi"("Enum"=enum16{"Read", "Write"}."Write", "error in (no error)"=w844, "I/P"=w828) -> ("error out"=w843:errorcluster)  [unwired: 7 in, 1 out]
              }
              frame True {
                w849 = i32[] [0, 0, 0, 0, 0]  # I/P
                n335 = call "PADMINI_AUTO_BARCODE_STATUS 60.vi"("Enum"=enum16{"Read", "Write"}."Write", "error in (no error)"=w853, "I/P"=w849) -> ("error out"=w852:errorcluster)  [unwired: 7 in, 1 out]
              }
            }
            n336 = flat-sequence {
              tunnel: [w856] -> w821
              tunnel: w822 -> [w856]
              frame #0 {
                # "UPDATE op 60 SCAN sTATUS"
                n337 = global write "DATA LOG.vi" "OP 60 Outputs"(TRUE) -> ()
              }
            }
          }
          frame "DATALOG6" {
            w870 = T15 2 items=["no dialog", "OK message", "continue or stop message", "OK message + warnings", "continue/stop + warnings"] ("type of dialog (OK msg:1)")
            # "datalog of OP 60"
            n338 = call "PADMINI_AUTO_BARCODE_STRING 60.vi"("Enum"=enum16{"Read", "Write"}."Read", "error in (no error)"=w862) -> ("error out"=w864:errorcluster, "Input 2"=w858:string[])  [unwired: 8 in]
            n339 = call "PADMINI_AUTO_CYCLE VALUE 60.vi"("Enum"=enum16{"Read", "Write"}."Read", "error in (no error)"=w862) -> ("Input 2"=w860:sgl[])  [unwired: 8 in, 1 out]
            n340 = Number To Fractional String(number=w860, precision (6)=i16 2) -> (F-format string=w859:string[])  [unwired: 2 in]
            n341 = case shown="False" w875 {
              tunnel: w876 -> [w903 w931]
              tunnel: w864 -> [w904 w930]
              tunnel: [w907 w929] -> w873
              tunnel: [w906 w928] -> w871
              tunnel: w874 -> [w902 _]
              tunnel: w859 -> [w898 w911]
              tunnel: w858 -> [w894 w910]
              frame False {
                # "DO TRACEBILITY"
                n342 = Index Array(array=w894) -> (element #1=w895:string, element #2=w886:string, element #3=w885:string, element #4=w884:string, element #5=w883:string, element #6=w882:string, element #7=w881:string, element #8=w880:string)  [unwired: 8 in]
                n343 = local read "SHIFT"() -> (w905:string)
                n344 = Index Array(array=w898) -> (element #1=w892:string, element #2=w891:string, element #3=w890:string, element #4=w889:string, element #5=w888:string, element #6=w887:string)  [unwired: 6 in]
                n345 = call <vilib>:"Trim Whitespace.vi"("string"=w895) -> ("trimmed string"=w896:string)  [unwired: 1 in]
                n346 = call "PADMINI_SHIFT_DATE.vi"("SHIFT"=w905) -> ("date/time string"=w893:string)  [unwired: 10 in]
                n347 = Format Into String(format string="Where BARCODE='%s' ", w896) -> (resulting string=w900:string)  [unwired: 2 in, 1 out]
                n348 = Bundle("date/time string"=w893, "Input 2"=w892, "Input 2"=w886, "Input 2"=w891, "Input 2"=w885, "Input 2"=w890, "Input 2"=w884, "Input 2"=w889, "Input 2"=w883, "Input 2"=w888, "Input 2"=w882, "Input 2"=w887, "Input 2"=w881, "Input 2"=w880) -> (w897:T25)  [unwired: 1 in]
                n349 = call <vilib>:"DB Tools Update Data.vi"("condition"=w900, "data"=w897, "error in (no error)"=w904, "columns"=string[] ["OP60_DATE", "OP60_SCREW1_DATA_Nm", "OP60_SCREW1_STATUS", "OP60_SCREW2_DATA_Nm", "OP60_SCREW2_STATUS", "OP60_SCREW3_DATA_Nm", "OP60_SCREW3_STATUS", "OP60_SCREW4_DATA_Nm", "OP60_SCREW4_STATUS", "OP60_SCREW5_DATA_Nm", "OP60_SCREW5_STATUS", "OP60_SCREW6_DATA_Nm", "OP60_SCREW6_STATUS", "OP60_FINAL_RESULT"], "table"=w902, "connection reference"=w903) -> ("error out"=w906:errorcluster, "connection reference out"=w907:T13)  [unwired: 4 in]
              }
              frame True {
                # "TRAC BYPASS"
                n350 = local read "SHIFT"() -> (w908:string)
                n351 = call "PADMINI_SHIFT_DATE.vi"("SHIFT"=w908) -> ("date/time string"=w909:string)  [unwired: 10 in]
                n352 = Index Array(array=w910) -> (element #2=w919:string, element #3=w918:string, element #4=w917:string, element #5=w915:string, element #6=w923:string, element #7=w924:string)  [unwired: 7 in, 1 out]
                n353 = Index Array(array=w911) -> (element #1=w922:string, element #2=w921:string, element #3=w920:string, element #4=w916:string, element #5=w914:string, element #6=w913:string)  [unwired: 6 in]
                n354 = Bundle("date/time string"=w909, "SHIFT"=w908, "Input 2"=w922, "Input 2"=w919, "Input 2"=w921, "Input 2"=w918, "Input 2"=w920, "Input 2"=w917, "Input 2"=w916, "Input 2"=w915, "Input 2"=w914, "Input 2"=w913, "Input 2"=w923, "Input 2"=w924) -> (w912:T26)  [unwired: 1 in]
                n355 = To Variant(anything=w912) -> (Variant=w927:variant)
                n356 = call <vilib>:"DB Tools Insert Data.vi"("data"=w927, "error in (no error)"=w930, "columns"=string[] ["DATE", "SHIFT", "ST6_SCREW1_DATA", "ST6_SCREW1_STATUS", "ST6_SCREW2_DATA", "ST6_SCREW2_STATUS", "ST6_SCREW3_DATA", "ST6_SCREW3_STATUS", "ST6_SCREW4_DATA", "ST6_SCREW4_STATUS", "ST6_SCREW5_DATA", "ST6_SCREW5_STATUS", "ST6_SCREW6_DATA", "ST6_SCREW6_STATUS", "ST6_FINAL_RST"], "table"="ST6_REPORT", "connection reference"=w931) -> ("error out"=w928:errorcluster, "connection reference out"=w929:T13)  [unwired: 5 in]
              }
            }
            n357 = call <vilib>:"Simple Error Handler.vi"("type of dialog (OK msg:1)"=w870, "error in (no error)"=w871) -> ("error out"=w869:errorcluster)  [unwired: 3 in, 4 out]
            n358 = call <vilib>:"Clear Errors.vi"("error in (no error)"=w869) -> ("error out"=w867:errorcluster)  [unwired: 5 in, 1 out]
            n359 = flat-sequence {
              tunnel: [w879] -> w857
              tunnel: w867 -> [w879]
              frame #0 {
                # "UPDATE op 20 save"
                n360 = global write "DATA LOG.vi" "OP 60 reset"(TRUE) -> ()
              }
            }
          }
          frame "SCAN7" {
            # "STATION OP 70"
            n361 = case shown="False" w938 {
              tunnel: w942 -> [w963 w969]
              tunnel: w941 -> [w956 w968]
              tunnel: w940 -> [w948 _]
              tunnel: [w958 w967] -> w937
              tunnel: [w957 w969] -> w939
              tunnel: [w949 "" ("trimmed string")] -> _
              frame False {
                n362 = call "PADMINI_AUTO_BARCODE_STRING 70.vi"("Enum"=enum16{"Read", "Write"}."Read", "error in (no error)"=w956) -> ("error out"=w955:errorcluster, "Input 2"=w951:string[])  [unwired: 8 in]
                n363 = Index Array(array=w951) -> (element=w950:string)  [unwired: 1 in]
                n364 = call <vilib>:"Trim Whitespace.vi"("string"=w950) -> ("trimmed string"=w949:string)  [unwired: 1 in]
                n365 = Format Into String(format string="WHERE BARCODE  ='%s'", w949) -> (resulting string=w952:string)  [unwired: 2 in, 1 out]
                n366 = call <vilib>:"DB Tools Select Data.vi"("condition"=w952, "error in (no error)"=w955, "columns"=string[] ["BARCODE", "OP60_FINAL_RESULT", "OP70_FINAL_RESULT"], "table"=w948, "connection reference"=w963) -> ("error out"=w961:errorcluster, "data"=w960:variant[][], "connection reference out"=w957:T13)  [unwired: 1 in]
                n367 = call "PADMINI_varient_to_data.vi"("error in (no error)"=w961, "data"=w960) -> ("error out"=w959:errorcluster, "Array"=w945:string[][])  [unwired: 8 in]
                n368 = Index Array(array=w945, index (row)=0 ("disabled index (col)")) -> (element=→"SCAN OP70":string[])  [unwired: 1 in]
                n369 = call "RESPONSE_LOGIC.vi"("Array"=w945) -> ("Not Found"=w943:i32[])  [unwired: 10 in]
                "OP70 STATUS" <- w943
                n370 = call "PADMINI_AUTO_BARCODE_STATUS 70.vi"("Enum"=enum16{"Read", "Write"}."Write", "error in (no error)"=w959, "I/P"=w943) -> ("error out"=w958:errorcluster)  [unwired: 7 in, 1 out]
              }
              frame True {
                w964 = i32[] [0, 0, 0, 0, 0]  # I/P
                n371 = call "PADMINI_AUTO_BARCODE_STATUS 70.vi"("Enum"=enum16{"Read", "Write"}."Write", "error in (no error)"=w968, "I/P"=w964) -> ("error out"=w967:errorcluster)  [unwired: 7 in, 1 out]
              }
            }
            n372 = flat-sequence {
              tunnel: [w971] -> w936
              tunnel: w937 -> [w971]
              frame #0 {
                # "UPDATE op 70 SCAN sTATUS"
                n373 = global write "DATA LOG.vi" "OP 70 Outputs"(TRUE) -> ()
              }
            }
          }
          frame "DATALOG7" {
            # "datalog of OP 70"
            n374 = call "PADMINI_AUTO_BARCODE_STRING 70.vi"("Enum"=enum16{"Read", "Write"}."Read", "error in (no error)"=w977) -> ("error out"=w979:errorcluster, "Input 2"=w973:string[])  [unwired: 8 in]
            n375 = call "PADMINI_AUTO_CYCLE VALUE 70.vi"("Enum"=enum16{"Read", "Write"}."Read", "error in (no error)"=w977) -> ("Input 2"=w975:sgl[])  [unwired: 8 in, 1 out]
            n376 = Number To Fractional String(number=w975, precision (6)=i16 4) -> (F-format string=w974:string[])  [unwired: 2 in]
            n377 = case shown="False" w987 {
              tunnel: w988 -> [w1006 w1024]
              tunnel: w979 -> [w1007 w1023]
              tunnel: [w1009 w1022] -> w985
              tunnel: [w1008 w1021] -> w983
              tunnel: w986 -> [w1005 _]
              tunnel: w974 -> [w1001 w1011]
              tunnel: w973 -> [w996 w1010]
              frame False {
                # "DO TRACEBILITY"
                n378 = Index Array(array=w996) -> (element #1=w997:string, element #2=w995:string)  [unwired: 2 in]
                n379 = call <vilib>:"Trim Whitespace.vi"("string"=w997) -> ("trimmed string"=w998:string)  [unwired: 1 in]
                n380 = local read "SHIFT"() -> (w993:string)
                n381 = Index Array(array=w1001) -> (element #1=w1000:string, element #2=w994:string)  [unwired: 2 in]
                n382 = call "PADMINI_SHIFT_DATE.vi"("SHIFT"=w993) -> ("date/time string"=w992:string)  [unwired: 10 in]
                n383 = Bundle("date/time string"=w992, "Input 2"=w1000, "Input 2"=w994, "Input 2"=w995) -> (w999:T27)  [unwired: 1 in]
                n384 = Format Into String(format string="Where BARCODE='%s' ", w998) -> (resulting string=w1003:string)  [unwired: 2 in, 1 out]
                n385 = call <vilib>:"DB Tools Update Data.vi"("condition"=w1003, "data"=w999, "error in (no error)"=w1007, "columns"=string[] ["OP70_DATE", "OP70_FULL_OPEN", "OP70_FULL_CLOSE", "OP70_FINAL_RESULT"], "table"=w1005, "connection reference"=w1006) -> ("error out"=w1008:errorcluster, "connection reference out"=w1009:T13)  [unwired: 4 in]
              }
              frame True {
                # "TRAC BYPASS"
                n386 = local read "SHIFT"() -> (w1012:string)
                n387 = call "PADMINI_SHIFT_DATE.vi"("SHIFT"=w1012) -> ("date/time string"=w1013:string)  [unwired: 10 in]
                n388 = Index Array(array=w1010) -> (element #2=w1016:string)  [unwired: 2 in, 1 out]
                n389 = Index Array(array=w1011) -> (element #1=w1017:string, element #2=w1015:string)  [unwired: 2 in]
                n390 = Bundle("date/time string"=w1013, "SHIFT"=w1012, "Input 2"=w1017, "Input 2"=w1015, "Input 2"=w1016) -> (w1014:T28)  [unwired: 1 in]
                n391 = To Variant(anything=w1014) -> (Variant=w1020:variant)
                n392 = call <vilib>:"DB Tools Insert Data.vi"("data"=w1020, "error in (no error)"=w1023, "columns"=string[] ["DATE_OP70", "SHIFT", "OP70_FULL_OPEN", "OP70_FULL_CLOSE", "OP70_FINAL_RST"], "table"="ST7_REPORT", "connection reference"=w1024) -> ("error out"=w1021:errorcluster, "connection reference out"=w1022:T13)  [unwired: 5 in]
              }
            }
            n393 = flat-sequence {
              tunnel: [w991] -> w972
              tunnel: w983 -> [w991]
              frame #0 {
                # "UPDATE op 20 save"
                n394 = global write "DATA LOG.vi" "OP 70 reset"(TRUE) -> ()
              }
            }
          }
          frame "SCAN8" {
            # "STATION OP 80"
            n395 = case shown="False" w1031 {
              tunnel: w1035 -> [w1056 w1062]
              tunnel: w1034 -> [w1049 w1061]
              tunnel: w1033 -> [w1041 _]
              tunnel: [w1051 w1060] -> w1030
              tunnel: [w1050 w1062] -> w1032
              tunnel: [w1042 "" ("trimmed string")] -> _
              frame False {
                (unwired) "REPORT"
                n396 = call "PADMINI_AUTO_BARCODE_STRING 80.vi"("Enum"=enum16{"Read", "Write"}."Read", "error in (no error)"=w1049) -> ("error out"=w1048:errorcluster, "Input 2"=w1044:string[])  [unwired: 8 in]
                n397 = Index Array(array=w1044) -> (element=w1043:string)  [unwired: 1 in]
                n398 = call <vilib>:"Trim Whitespace.vi"("string"=w1043) -> ("trimmed string"=w1042:string)  [unwired: 1 in]
                n399 = Format Into String(format string="WHERE BARCODE  ='%s'", w1042) -> (resulting string=w1045:string)  [unwired: 2 in, 1 out]
                n400 = call <vilib>:"DB Tools Select Data.vi"("condition"=w1045, "error in (no error)"=w1048, "columns"=string[] ["BARCODE", "OP70_FINAL_RESULT", "OP80_FINAL_RESULT"], "table"=w1041, "connection reference"=w1056) -> ("error out"=w1054:errorcluster, "data"=w1053:variant[][], "connection reference out"=w1050:T13)  [unwired: 1 in]
                n401 = call "PADMINI_varient_to_data.vi"("error in (no error)"=w1054, "data"=w1053) -> ("error out"=w1052:errorcluster, "Array"=w1038:string[][])  [unwired: 8 in]
                n402 = Index Array(array=w1038, index (row)=0 ("disabled index (col)")) -> (element=→"SCAN OP80":string[])  [unwired: 1 in]
                n403 = call "RESPONSE_LOGIC.vi"("Array"=w1038) -> ("Not Found"=w1037:i32[])  [unwired: 10 in]
                "OP80 STATUS" <- w1037
                n404 = call "PADMINI_AUTO_BARCODE_STATUS 80.vi"("Enum"=enum16{"Read", "Write"}."Write", "error in (no error)"=w1052, "I/P"=w1037) -> ("error out"=w1051:errorcluster)  [unwired: 7 in, 1 out]
              }
              frame True {
                w1057 = i32[] [0, 0, 0, 0, 0]  # I/P
                n405 = call "PADMINI_AUTO_BARCODE_STATUS 80.vi"("Enum"=enum16{"Read", "Write"}."Write", "error in (no error)"=w1061, "I/P"=w1057) -> ("error out"=w1060:errorcluster)  [unwired: 7 in, 1 out]
              }
            }
            n406 = flat-sequence {
              tunnel: [w1064] -> w1029
              tunnel: w1030 -> [w1064]
              frame #0 {
                # "UPDATE op 80 SCAN sTATUS"
                n407 = global write "DATA LOG.vi" "OP 80 Outputs"(TRUE) -> ()
              }
            }
          }
          frame "DATALOG8" {
            w1079 = T15 2 items=["no dialog", "OK message", "continue or stop message", "OK message + warnings", "continue/stop + warnings"] ("type of dialog (OK msg:1)")
            # "datalog of OP 80"
            n408 = call "PADMINI_AUTO_BARCODE_STRING 80.vi"("Enum"=enum16{"Read", "Write"}."Read", "error in (no error)"=w1071) -> ("error out"=w1073:errorcluster, "Input 2"=w1067:string[])  [unwired: 8 in]
            n409 = call "PADMINI_AUTO_CYCLE VALUE 80.vi"("Enum"=enum16{"Read", "Write"}."Read", "error in (no error)"=w1071) -> ("Input 2"=w1069:sgl[])  [unwired: 8 in, 1 out]
            n410 = Number To Fractional String(number=w1069, precision (6)=i16 2) -> (F-format string=w1068:string[])  [unwired: 2 in]
            n411 = case shown="True" w1065 {
              tunnel: w1084 -> [w1102 w1121]
              tunnel: w1073 -> [w1103 w1120]
              tunnel: [w1105 w1119] -> w1082
              tunnel: [w1104 w1118] -> w1080
              tunnel: w1083 -> [w1101 w1106]
              tunnel: w1068 -> [w1097 w1111]
              tunnel: w1067 -> [w1093 w1112]
              frame False {
                # "DO TRACEBILITY"
                n412 = Index Array(array=w1093) -> (element #1=w1094:string, element #2=w1089:string, element #3=w1088:string)  [unwired: 3 in]
                n413 = call <vilib>:"Trim Whitespace.vi"("string"=w1094) -> ("trimmed string"=w1095:string)  [unwired: 1 in]
                n414 = local read "SHIFT"() -> (w1092:string)
                n415 = Index Array(array=w1097) -> (element=w1090:string)  [unwired: 1 in]
                n416 = call "PADMINI_SHIFT_DATE.vi"("SHIFT"=w1092) -> ("date/time string"=w1091:string)  [unwired: 10 in]
                n417 = Bundle("date/time string"=w1091, "Input 2"=w1089, "Input 2"=w1090, "Input 2"=w1088) -> (w1096:T27)  [unwired: 1 in]
                n418 = Format Into String(format string="Where BARCODE='%s' ", w1095) -> (resulting string=w1099:string)  [unwired: 2 in, 1 out]
                n419 = call <vilib>:"DB Tools Update Data.vi"("condition"=w1099, "data"=w1096, "error in (no error)"=w1103, "columns"=string[] ["OP80_DATE", "OP80_LOCTITE_STATUS", "OP80_PLUG_PRESS_LOAD_kg", "OP80_FINAL_RESULT"], "table"=w1101, "connection reference"=w1102) -> ("error out"=w1104:errorcluster, "connection reference out"=w1105:T13)  [unwired: 4 in]
              }
              frame True {
                (unwired) "ST8_REPORT"
                # "TRAC BYPASS"
                n420 = local read "SHIFT"() -> (w1108:string)
                n421 = call "PADMINI_SHIFT_DATE.vi"("SHIFT"=w1108) -> ("date/time string"=w1107:string)  [unwired: 10 in]
                n422 = Index Array(array=w1112) -> (element #1=w1109:string, element #2=w1116:string, element #3=w1115:string)  [unwired: 3 in]
                n423 = Index Array(array=w1111) -> (element=w1114:string)  [unwired: 1 in]
                n424 = Bundle("Input 2"=w1109, "SHIFT"=w1108, "date/time string"=w1107, "Input 2"=w1114, "Input 2"=w1116, "Input 2"=w1115) -> (w1113:T29)  [unwired: 1 in]
                n425 = To Variant(anything=w1113) -> (Variant=w1117:variant)
                n426 = call <vilib>:"DB Tools Insert Data.vi"("data"=w1117, "error in (no error)"=w1120, "columns"=string[] ["BARCODE", "SHIFT", "OP80_DATE", "OP80_LOCTITE_STATUS", "OP80_PLUG_PRESS_LOAD_kg", "OP80_FINAL_RESULT"], "table"=w1106, "connection reference"=w1121) -> ("error out"=w1118:errorcluster, "connection reference out"=w1119:T13)  [unwired: 5 in]
              }
            }
            n427 = call <vilib>:"Simple Error Handler.vi"("type of dialog (OK msg:1)"=w1079, "error in (no error)"=w1080) -> ("error out"=w1078:errorcluster)  [unwired: 3 in, 4 out]
            n428 = call <vilib>:"Clear Errors.vi"("error in (no error)"=w1078) -> ("error out"=w1076:errorcluster)  [unwired: 5 in, 1 out]
            n429 = flat-sequence {
              tunnel: [w1087] -> w1066
              tunnel: w1076 -> [w1087]
              frame #0 {
                # "UPDATE op 20 save"
                n430 = global write "DATA LOG.vi" "OP 80 reset"(TRUE) -> ()
              }
            }
          }
          frame "SCAN9" {
            # "STATION OP 90"
            n431 = case shown="False" w1128 {
              tunnel: w1132 -> [w1153 w1159]
              tunnel: w1131 -> [w1146 w1158]
              tunnel: w1130 -> [w1138 _]
              tunnel: [w1148 w1157] -> w1127
              tunnel: [w1147 w1159] -> w1129
              tunnel: [w1139 "" ("trimmed string")] -> _
              frame False {
                (unwired) "REPORT"
                n432 = call "PADMINI_AUTO_BARCODE_STRING 90.vi"("Enum"=enum16{"Read", "Write"}."Read", "error in (no error)"=w1146) -> ("error out"=w1145:errorcluster, "Input 2"=w1141:string[])  [unwired: 8 in]
                n433 = Index Array(array=w1141) -> (element=w1140:string)  [unwired: 1 in]
                n434 = call <vilib>:"Trim Whitespace.vi"("string"=w1140) -> ("trimmed string"=w1139:string)  [unwired: 1 in]
                n435 = Format Into String(format string="WHERE BARCODE  ='%s'", w1139) -> (resulting string=w1142:string)  [unwired: 2 in, 1 out]
                n436 = call <vilib>:"DB Tools Select Data.vi"("condition"=w1142, "error in (no error)"=w1145, "columns"=string[] ["BARCODE", "OP80_FINAL_RESULT", "OP90_FINAL_RESULT"], "table"=w1138, "connection reference"=w1153) -> ("error out"=w1151:errorcluster, "data"=w1150:variant[][], "connection reference out"=w1147:T13)  [unwired: 1 in]
                n437 = call "PADMINI_varient_to_data.vi"("error in (no error)"=w1151, "data"=w1150) -> ("error out"=w1149:errorcluster, "Array"=w1135:string[][])  [unwired: 8 in]
                n438 = Index Array(array=w1135, index (row)=0 ("disabled index (col)")) -> (element=→"SCAN OP90":string[])  [unwired: 1 in]
                n439 = call "RESPONSE_LOGIC.vi"("Array"=w1135) -> ("Not Found"=w1133:i32[])  [unwired: 10 in]
                "OP90 STATUS" <- w1133
                n440 = call "PADMINI_AUTO_BARCODE_STATUS 90.vi"("Enum"=enum16{"Read", "Write"}."Write", "error in (no error)"=w1149, "I/P"=w1133) -> ("error out"=w1148:errorcluster)  [unwired: 7 in, 1 out]
              }
              frame True {
                w1154 = i32[] [0, 0, 0, 0, 0]  # I/P
                n441 = call "PADMINI_AUTO_BARCODE_STATUS 90.vi"("Enum"=enum16{"Read", "Write"}."Write", "error in (no error)"=w1158, "I/P"=w1154) -> ("error out"=w1157:errorcluster)  [unwired: 7 in, 1 out]
              }
            }
            n442 = flat-sequence {
              tunnel: [w1161] -> w1126
              tunnel: w1127 -> [w1161]
              frame #0 {
                # "UPDATE op 90 SCAN sTATUS"
                n443 = global write "DATA LOG.vi" "OP 90 Outputs"(TRUE) -> ()
              }
            }
          }
          frame "DATALOG9" {
            w1175 = T15 2 items=["no dialog", "OK message", "continue or stop message", "OK message + warnings", "continue/stop + warnings"] ("type of dialog (OK msg:1)")
            # "datalog of OP 90"
            n444 = call "PADMINI_AUTO_BARCODE_STRING 90.vi"("Enum"=enum16{"Read", "Write"}."Read", "error in (no error)"=w1167) -> ("error out"=w1169:errorcluster, "Input 2"=w1164:string[])  [unwired: 8 in]
            n445 = call "PADMINI_AUTO_CYCLE VALUE 90.vi"("Enum"=enum16{"Read", "Write"}."Read", "error in (no error)"=w1167) -> ("Input 2"=w1163:sgl[])  [unwired: 8 in, 1 out]
            n446 = Number To Fractional String(number=w1163, precision (6)=i16 2) -> (F-format string=w1165:string[])  [unwired: 2 in]
            n447 = case shown="False" w1180 {
              tunnel: w1181 -> [w1200 w1219]
              tunnel: w1169 -> [w1201 w1218]
              tunnel: [w1203 w1217] -> w1178
              tunnel: [w1202 w1216] -> w1176
              tunnel: w1179 -> [w1199 _]
              tunnel: w1165 -> [w1195 w1208]
              tunnel: w1164 -> [w1191 w1207]
              frame False {
                # "DO TRACEBILITY"
                n448 = Index Array(array=w1191) -> (element #1=w1192:string, element #2=w1189:string, element #3=w1187:string)  [unwired: 3 in]
                n449 = call <vilib>:"Trim Whitespace.vi"("string"=w1192) -> ("trimmed string"=w1193:string)  [unwired: 1 in]
                n450 = local read "SHIFT"() -> (w1186:string)
                n451 = Index Array(array=w1195) -> (element #1=w1190:string, element #2=w1188:string)  [unwired: 2 in]
                n452 = call "PADMINI_SHIFT_DATE.vi"("SHIFT"=w1186) -> ("date/time string"=w1185:string)  [unwired: 10 in]
                n453 = Bundle("date/time string"=w1185, "Input 2"=w1190, "Input 2"=w1189, "Input 2"=w1188, "Input 2"=w1187) -> (w1194:T20)  [unwired: 1 in]
                n454 = Format Into String(format string="Where BARCODE='%s' ", w1193) -> (resulting string=w1197:string)  [unwired: 2 in, 1 out]
                n455 = call <vilib>:"DB Tools Update Data.vi"("condition"=w1197, "data"=w1194, "error in (no error)"=w1201, "columns"=string[] ["OP90_DATE", "OP90_SEAT_LEAK_LP", "OP90_SEAT_STATUS", "OP90_STEAM_LEAK_sccm", "OP90_FINAL_RESULT"], "table"=w1199, "connection reference"=w1200) -> ("error out"=w1202:errorcluster, "connection reference out"=w1203:T13)  [unwired: 4 in]
              }
              frame True {
                # "TRAC BYPASS"
                n456 = local read "SHIFT"() -> (w1204:string)
                n457 = call "PADMINI_SHIFT_DATE.vi"("SHIFT"=w1204) -> ("date/time string"=w1205:string)  [unwired: 10 in]
                n458 = Index Array(array=w1207) -> (element #2=w1212:string, element #3=w1210:string)  [unwired: 3 in, 1 out]
                n459 = Index Array(array=w1208) -> (element #1=w1213:string, element #2=w1211:string)  [unwired: 2 in]
                n460 = Bundle("date/time string"=w1205, "SHIFT"=w1204, "Input 2"=w1213, "Input 2"=w1212, "Input 2"=w1211, "Input 2"=w1210) -> (w1209:T21)  [unwired: 1 in]
                n461 = To Variant(anything=w1209) -> (Variant=w1215:variant)
                n462 = call <vilib>:"DB Tools Insert Data.vi"("data"=w1215, "error in (no error)"=w1218, "columns"=string[] ["DATE", "SHIFT", "ST9_SEAT_LT_DATA", "ST9_SEAT_STATUS", "ST9_STEAM_LT_DATA", "ST9_FINAL_RST"], "table"="ST9_REPORT", "connection reference"=w1219) -> ("error out"=w1216:errorcluster, "connection reference out"=w1217:T13)  [unwired: 5 in]
              }
            }
            n463 = call <vilib>:"Simple Error Handler.vi"("type of dialog (OK msg:1)"=w1175, "error in (no error)"=w1176) -> ("error out"=w1174:errorcluster)  [unwired: 3 in, 4 out]
            n464 = call <vilib>:"Clear Errors.vi"("error in (no error)"=w1174) -> ("error out"=w1172:errorcluster)  [unwired: 5 in, 1 out]
            n465 = flat-sequence {
              tunnel: [w1184] -> w1162
              tunnel: w1172 -> [w1184]
              frame #0 {
                # "UPDATE op 20 save"
                n466 = global write "DATA LOG.vi" "OP 90 reset"(TRUE) -> ()
              }
            }
          }
          frame "SCAN10" {
            # "STATION OP 10"
            n467 = case shown="False" w1226 {
              tunnel: w1230 -> [w1251 w1257]
              tunnel: w1229 -> [w1245 w1256]
              tunnel: w1228 -> [w1237 _]
              tunnel: [w1235 w1255] -> w1225
              tunnel: [w1246 w1257] -> w1227
              tunnel: [w1238 "" ("trimmed string")] -> _
              frame False {
                (unwired) "REPORT"
                n468 = call "PADMINI_AUTO_BARCODE_STRING 100.vi"("Enum"=enum16{"Read", "Write"}."Read", "error in (no error)"=w1245) -> ("error out"=w1244:errorcluster, "Input 2"=w1240:string[])  [unwired: 8 in]
                n469 = Index Array(array=w1240) -> (element=w1239:string)  [unwired: 1 in]
                n470 = call <vilib>:"Trim Whitespace.vi"("string"=w1239) -> ("trimmed string"=w1238:string)  [unwired: 1 in]
                n471 = Format Into String(format string="WHERE BARCODE  ='%s'", w1238) -> (resulting string=w1241:string)  [unwired: 2 in, 1 out]
                n472 = call <vilib>:"DB Tools Select Data.vi"("condition"=w1241, "error in (no error)"=w1244, "columns"=string[] ["BARCODE", "OP90_FINAL_RESULT", "OP100_FINAL_RESULT"], "table"=w1237, "connection reference"=w1251) -> ("error out"=w1249:errorcluster, "data"=w1248:variant[][], "connection reference out"=w1246:T13)  [unwired: 1 in]
                n473 = call "PADMINI_varient_to_data.vi"("error in (no error)"=w1249, "data"=w1248) -> ("error out"=w1247:errorcluster, "Array"=w1233:string[][])  [unwired: 8 in]
                n474 = Index Array(array=w1233, index (row)=0 ("disabled index (col)")) -> (element=→"SCAN OP100":string[])  [unwired: 1 in]
                n475 = call "RESPONSE_LOGIC.vi"("Array"=w1233) -> ("Not Found"=w1231:i32[])  [unwired: 10 in]
                "OP100 STATUS" <- w1231
                n476 = call "PADMINI_AUTO_BARCODE_STATUS 100.vi"("Enum"=enum16{"Read", "Write"}."Write", "error in (no error)"=w1247, "I/P"=w1231) -> ("error out"=w1235:errorcluster)  [unwired: 7 in, 1 out]
              }
              frame True {
                w1252 = i32[] [0, 0, 0, 0, 0]  # I/P
                n477 = call "PADMINI_AUTO_BARCODE_STATUS 100.vi"("Enum"=enum16{"Read", "Write"}."Write", "error in (no error)"=w1256, "I/P"=w1252) -> ("error out"=w1255:errorcluster)  [unwired: 7 in, 1 out]
              }
            }
            n478 = flat-sequence {
              tunnel: [w1259] -> w1224
              tunnel: w1225 -> [w1259]
              frame #0 {
                # "UPDATE op 100 SCAN sTATUS"
                n479 = global write "DATA LOG.vi" "OP 100 Outputs"(TRUE) -> ()
              }
            }
          }
          frame "SCAN11" {
            # "STATION OP 110"
            n480 = case shown="False" w1266 {
              tunnel: w1270 -> [w1297 w1307]
              tunnel: w1269 -> [w1290 w1306]
              tunnel: w1268 -> [w1282 _]
              tunnel: [w1292 w1305] -> w1265
              tunnel: [w1291 w1307] -> w1267
              frame False {
                (unwired) "REPORT"
                # "OP100 OK\nOP 100 NG"
                n481 = call "PADMINI_AUTO_BARCODE_STRING 100.vi"("Enum"=enum16{"Read", "Write"}."Read", "error in (no error)"=w1290) -> ("error out"=w1289:errorcluster, "Input 2"=w1284:string[])  [unwired: 8 in]
                n482 = Index Array(array=w1284) -> (element=w1283:string)  [unwired: 1 in]
                n483 = call <vilib>:"Trim Whitespace.vi"("string"=w1283) -> ("trimmed string"=w1285:string)  [unwired: 1 in]
                n484 = Format Into String(format string="WHERE BARCODE  ='%s'", w1285) -> (resulting string=w1286:string)  [unwired: 2 in, 1 out]
                n485 = call <vilib>:"DB Tools Select Data.vi"("condition"=w1286, "error in (no error)"=w1289, "columns"=string[] ["BARCODE", "OP100_FINAL_RESULT"], "table"=w1282, "connection reference"=w1297) -> ("error out"=w1295:errorcluster, "data"=w1294:variant[][], "connection reference out"=w1291:T13)  [unwired: 1 in]
                n486 = call "PADMINI_varient_to_data.vi"("error in (no error)"=w1295, "data"=w1294) -> ("error out"=w1293:errorcluster, "Array"=w1273:string[][])  [unwired: 8 in]
                n487 = Index Array(array=w1273, index (row)=0 ("disabled index (col)")) -> (element=w1272:string[])  [unwired: 1 in]
                "SCAN OP110" <- w1272
                n488 = Index Array(array=w1272) -> (element #1=w1280:string, element #2=w1277:string)  [unwired: 2 in]
                n489 = Equal?(x="", y=w1280) -> (x = y?=w1279:bool)
                n490 = Equal?(x=w1277, y="OK") -> (x = y?=w1278:bool)
                n491 = case shown="True" w1279 {
                  tunnel: w1278 -> [w1298 _]
                  tunnel: [w1299 w1302] -> w1271
                  frame False {
                    # "BARCODE FOUND"
                    n492 = case shown="False" w1298 {
                      tunnel: [w1300 w1301] -> w1299
                      frame False {
                        w1300 = i32[] [0, 1]  # OK
                        # "CT ST REPEAT NG & EMPTY"
                      }
                      frame True {
                        w1301 = i32[] [1, 0]  # NG
                        # "CT ST REPEAT EMPTY"
                      }
                    }
                  }
                  frame True {
                    w1302 = i32[] [0, 1]  # Not Found
                    # "nO BARCODE FOUND"
                  }
                }
                "OP110 STATUS" <- w1271
                n493 = call "PADMINI_AUTO_BARCODE_STATUS 110.vi"("Enum"=enum16{"Read", "Write"}."Write", "error in (no error)"=w1293, "I/P"=w1271) -> ("error out"=w1292:errorcluster)  [unwired: 7 in, 1 out]
              }
              frame True {
                w1303 = i32[] [0, 0, 0, 0, 0]  # I/P
                n494 = call "PADMINI_AUTO_BARCODE_STATUS 100.vi"("Enum"=enum16{"Read", "Write"}."Write", "error in (no error)"=w1306, "I/P"=w1303) -> ("error out"=w1305:errorcluster)  [unwired: 7 in, 1 out]
              }
            }
            n495 = flat-sequence {
              tunnel: [w1309] -> w1264
              tunnel: w1265 -> [w1309]
              frame #0 {
                # "UPDATE op 100 SCAN sTATUS"
                n496 = global write "DATA LOG.vi" "OP 110 Outputs"(TRUE) -> ()
              }
            }
          }
          frame "DATALOG10" {
            w1323 = T15 2 items=["no dialog", "OK message", "continue or stop message", "OK message + warnings", "continue/stop + warnings"] ("type of dialog (OK msg:1)")
            # "datalog of OP 100"
            n497 = call "PADMINI_AUTO_BARCODE_STRING 100.vi"("Enum"=enum16{"Read", "Write"}."Read", "error in (no error)"=w1311) -> ("error out"=w1317:errorcluster, "Input 2"=w1313:string[])  [unwired: 8 in]
            n498 = call "PADMINI_AUTO_CYCLE VALUE 100.vi"("Enum"=enum16{"Read", "Write"}."Read", "error in (no error)"=w1311) -> ("Input 2"=w1312:sgl[])  [unwired: 8 in, 1 out]
            n499 = Number To Fractional String(number=w1312, precision (6)=i16 2) -> (F-format string=w1314:string[])  [unwired: 2 in]
            n500 = case shown="False" w1328 {
              tunnel: w1329 -> [w1357 w1382]
              tunnel: w1317 -> [w1358 w1381]
              tunnel: [w1360 w1380] -> w1326
              tunnel: [w1359 w1379] -> w1324
              tunnel: w1327 -> [w1356 _]
              tunnel: w1314 -> [w1352 w1364]
              tunnel: w1313 -> [w1349 w1365]
              frame False {
                # "DO TRACEBILITY"
                n501 = Index Array(array=w1349) -> (element #1=w1348:string, element #2=w1334:string, element #3=w1333:string)  [unwired: 3 in]
                n502 = call <vilib>:"Trim Whitespace.vi"("string"=w1348) -> ("trimmed string"=w1350:string)  [unwired: 1 in]
                n503 = Index Array(array=w1352) -> (element #1=w1345:string, element #2=w1344:string, element #3=w1343:string, element #4=w1342:string, element #5=w1341:string, element #6=w1340:string, element #7=w1339:string, element #8=w1338:string, element #9=w1337:string, element #10=w1336:string, element #11=w1335:string)  [unwired: 11 in]
                n504 = local read "SHIFT"() -> (w1347:string)
                n505 = call "PADMINI_SHIFT_DATE.vi"("SHIFT"=w1347) -> ("date/time string"=w1346:string)  [unwired: 10 in]
                n506 = Bundle("date/time string"=w1346, "Input 2"=w1345, "Input 2"=w1344, "Input 2"=w1343, "Input 2"=w1342, "Input 2"=w1341, "Input 2"=w1340, "Input 2"=w1339, "Input 2"=w1338, "Input 2"=w1337, "Input 2"=w1336, "Input 2"=w1335, "Input 2"=w1334, "Input 2"=w1333) -> (w1351:T25)  [unwired: 1 in]
                n507 = Format Into String(format string="Where BARCODE='%s' ", w1350) -> (resulting string=w1354:string)  [unwired: 2 in, 1 out]
                n508 = call <vilib>:"DB Tools Update Data.vi"("condition"=w1354, "data"=w1351, "error in (no error)"=w1358, "columns"=string[] ["OP100_DATE", "OP100_SENSOR_OP_OPEN_V", "OP100_SENSOR_OP_CLOSE_V", "OP100_SENSOR_OP_FULL_CLOSE_V", "OP100_SENSOR_INITIAL_V", "OP100_MOTOR_START_OF_CLOSE_V", "OP100_MOTOR_FULL_CLOSE_V", "OP100_MOTOR_START_BACK_V", "OP100_MOTOR_FULL_OPEN_V", "OP100_RESPONSE_TIME_FWD_msec", "OP100_RESPONSE_TIME_REV_msec", "OP100_MOTOR_PEAK_CURRENT_A", "OP100_FINAL_RESULT", "OP100_CONNECTOR_CAMERA_STATUS"], "table"=w1356, "connection reference"=w1357) -> ("error out"=w1359:errorcluster, "connection reference out"=w1360:T13)  [unwired: 4 in]
              }
              frame True {
                # "TRAC BYPASS"
                n509 = local read "SHIFT"() -> (w1362:string)
                n510 = Index Array(array=w1365) -> (element=w1369:string)  [unwired: 1 in]
                n511 = call "PADMINI_SHIFT_DATE.vi"("SHIFT"=w1362) -> ("date/time string"=w1363:string)  [unwired: 10 in]
                n512 = Index Array(array=w1364) -> (element #1=w1375:string, element #2=w1374:string, element #3=w1361:string, element #4=w1367:string, element #5=w1373:string, element #6=w1368:string, element #7=w1372:string, element #8=w1371:string, element #9=w1370:string)  [unwired: 9 in]
                n513 = Bundle("date/time string"=w1363, "SHIFT"=w1362, "Input 2"=w1375, "Input 2"=w1374, "Input 2"=w1361, "Input 2"=w1361, "Input 2"=w1361, "Input 2"=w1367, "Input 2"=w1373, "Input 2"=w1368, "Input 2"=w1372, "Input 2"=w1371, "Input 2"=w1370, "Input 2"=w1369) -> (w1366:T26)  [unwired: 1 in]
                n514 = To Variant(anything=w1366) -> (Variant=w1378:variant)
                n515 = call <vilib>:"DB Tools Insert Data.vi"("data"=w1378, "error in (no error)"=w1381, "columns"=string[] ["DATE", "SHIFT", "ST10_SENSOR_OP_OPEN_V", "ST10_START_OF_CLOSE_SENSOR_V", "ST10_SENSOR_OP_FULL_CLOSE_V", "ST10_RESPONSE_TIME_FWD", "ST10_RESPONSE_TIME_REV", "ST10_MOTOR_V_START_OF_CLOSE_A", "ST10_MOTOR_V_FULL_CLOSE_B", "ST10_MOTOR_V_START_BACK_C", "ST10_MOTOR_V_FULL_OPEN_D", "ST10_MOTOR_RMS_CURRENT_A", "ST10_FINAL_RST"], "table"="ST10_REPORT", "connection reference"=w1382) -> ("error out"=w1379:errorcluster, "connection reference out"=w1380:T13)  [unwired: 5 in]
              }
            }
            n516 = call <vilib>:"Simple Error Handler.vi"("type of dialog (OK msg:1)"=w1323, "error in (no error)"=w1324) -> ("error out"=w1322:errorcluster)  [unwired: 3 in, 4 out]
            n517 = call <vilib>:"Clear Errors.vi"("error in (no error)"=w1322) -> ("error out"=w1320:errorcluster)  [unwired: 5 in, 1 out]
            n518 = flat-sequence {
              tunnel: [w1332] -> w1310
              tunnel: w1320 -> [w1332]
              frame #0 {
                # "UPDATE op 20 save"
                n519 = global write "DATA LOG.vi" "OP 100 reset"(TRUE) -> ()
              }
            }
          }
          frame "EMERGENCY STOP" {
          }
          frame "STOP" {
            n520 = global read "Global 1.vi" "BARCODE RECIPE"() -> (w1393:string)
            n521 = Bundle("BARCODE RECIPE"=w1393) -> (w1392:cluster{"BARCODE RECIPE":string})  [unwired: 1 in]
            n522 = call <vilib>:"DB Tools Update Data.vi"("data"=w1392, "error in (no error)"=w1398, "columns"=string[] ["PREVIOUS_LOADED_RECIPE"], "table"="BARCODE_RECIPE", "connection reference"=w1396) -> ("error out"=w1397:errorcluster, "connection reference out"=w1395:T13)  [unwired: 5 in]
          }
        }
      }
      frame Error {
        # "Return true in any case that should stop the loop."
      }
    }
    n523 = Unbundle By Name(w130) -> ("OP - 90"=→"OP - 90":T30, "OP - 100"=→"OP - 100":T10, "OP - 110"=→"OP - 110":cluster{"BARCODE":string})
    n524 = Unbundle By Name(w130) -> ("OP - 10"=→"OP - 10":T31, "OP - 20"=→"OP - 20":T5, "OP - 30"=→"OP - 30":T32, "OP - 40"=→"OP - 40":T2)
    n525 = Unbundle By Name(w130) -> ("OP - 50"=→"OP - 50":T1, "OP - 60"=→"OP - 60":T33, "OP - 70"=→"OP - 70":T34, "OP - 80"=→"OP - 80":T35)
    n526 = Wait (ms)(milliseconds to wait=u32 100) -> ()  [unwired: 1 out]
    n527 = call <vilib>:"Simple Error Handler.vi"("error in (no error)"=w124) -> ("error out"=w123:errorcluster)  [unwired: 4 in, 4 out]
  }
  n528 = while {
    shift-right: [w1422] -> w72
    shift-left: w22 -> [w1416]
    shift-right: [w1423] -> w66
    shift-left: w70 -> [w1431]
    stop <- w1421 stop-if-true
    n529 = local read "Shift_change"() -> (w1429:bool)
    n530 = call <vilib>:"Clear Errors.vi"("error in (no error)"=w1416) -> ("error out"=w1407:errorcluster)  [unwired: 5 in, 1 out]
    n531 = call "READ EMERGENCY BIT.vi"("Enum"=enum16{"Read", "Write"}."Read", "error in (no error)"=w1407) -> ("Array Out"=w1419:dbl[])  [unwired: 8 in, 1 out]
    n532 = case shown="True" w1429 {
      tunnel: w1407 -> [w1448 w1461]
      tunnel: [w1449 w1460] -> w1428
      frame False {
        n533 = local read "SHIFT_DATA 2"() -> (w1451:string[])
        n534 = Get Date/Time In Seconds() -> (seconds since 1Jan1904=w1450:timestamp)
        n535 = call "String To Time_4.vi"("error in (no error)"=w1448, "String Array In"=w1451) -> ("error out"=w1447:errorcluster, "Time Stamp Out"=w1446:timestamp[])  [unwired: 8 in]
        "Time Stamp Out 4" <- w1446
        n536 = call "Shift Calculation_4.vi"("error in (no error)"=w1447, "Current Time"=w1450, "Time Stamp Out"=w1446) -> ("error out"=w1445:errorcluster, "Shift"=w1444:i32)  [unwired: 7 in]
        n537 = call <vilib>:"Clear Errors.vi"("error in (no error)"=w1445) -> ()  [unwired: 5 in, 2 out]
        n538 = case shown="4" w1444 {
          tunnel: ["A" "B" "C" "D"] -> w1449
          frame 1, Default {
          }
          frame 2 {
          }
          frame 3 {
          }
          frame 4 {
          }
        }
      }
      frame True {
        n539 = local read "SHIFT_DATA"() -> (w1459:string[])
        n540 = Get Date/Time In Seconds() -> (seconds since 1Jan1904=w1462:timestamp)
        n541 = call "String To Time.vi"("error in (no error)"=w1461, "String Array In"=w1459) -> ("error out"=w1458:errorcluster, "Time Stamp Out"=w1463:timestamp[])  [unwired: 8 in]
        "Time Stamp Out" <- w1463
        n542 = call "Shift Calculation.vi"("error in (no error)"=w1458, "Current Time"=w1462, "Time Stamp Out"=w1463) -> ("error out"=w1457:errorcluster, "Shift"=w1456:i32)  [unwired: 7 in]
        "Shift 4" <- w1456
        n543 = call <vilib>:"Clear Errors.vi"("error in (no error)"=w1457) -> ()  [unwired: 5 in, 2 out]
        n544 = case shown="3" w1456 {
          tunnel: ["A" "B" "C"] -> w1460
          frame 1, Default {
          }
          frame 2 {
          }
          frame 3 {
          }
        }
      }
    }
    "SHIFT" <- w1428
    n545 = Index Array(array=w1419) -> (element=w1418:dbl)  [unwired: 1 in]
    n546 = call "VALUE_CHANGE - ST1_RESULT.vi"("Numeric"=w1418) -> ("Boolean"=w1417:bool)  [unwired: 9 in, 1 out]
    n547 = global write "Global 1.vi" "EMERGENCY STOP"(w1417) -> ()
    n548 = call "Trigger_Loggic.vi"("error in (no error)"=w1407) -> ("error out"=w1412:errorcluster, "Array"=w1432:i32[])  [unwired: 9 in]
    n549 = for {
      tunnel: w1432 -> [w1467] mode=indexing
      shift-right: [w1471] -> w1425
      shift-left: w1431 -> [w1470]
      shift-right: [w1469] -> w1424
      shift-left: w1412 -> [w1468]
      n550 = case shown="0" w1467 {
        tunnel: [w1474 w1479 w1483 w1489 w1494 w1499 w1504 w1509 w1514 w1519 w1524 w1529 w1534 w1539 w1544 w1549 w1554 w1559 w1564 w1569 w1574 w1579 w1584] -> w1471
        tunnel: w1470 -> [w1476 w1481 w1484 w1491 w1496 w1501 w1506 w1511 w1516 w1521 w1526 w1531 w1536 w1541 w1546 w1551 w1556 w1561 w1566 w1571 w1576 w1581 w1586]
        tunnel: [w1473 w1478 w1485 w1488 w1493 w1498 w1503 w1508 w1513 w1518 w1523 w1528 w1533 w1538 w1543 w1548 w1553 w1558 w1563 w1568 w1573 w1578 w1583] -> w1469
        tunnel: w1468 -> [w1475 w1480 w1486 w1490 w1495 w1500 w1505 w1510 w1515 w1520 w1525 w1530 w1535 w1540 w1545 w1550 w1555 w1560 w1565 w1570 w1575 w1580 w1585]
        frame -1, Default {
          # "DEFAULT"
          n551 = Enqueue Element(queue=w1476, element=cluster{"CASE 2":T12} {"CASE 2"=enum."-1"}, error in (no error)=w1475) -> (queue out=w1474:refnum<queue>, error out=w1473:errorcluster)  [unwired: 1 in, 1 out]
        }
        frame 0 {
          # "SCAN BARCODE OP 10"
          n552 = Enqueue Element(queue=w1481, element=cluster{"CASE 2":T12} {"CASE 2"=enum."-1"}, error in (no error)=w1480) -> (queue out=w1479:refnum<queue>, error out=w1478:errorcluster)  [unwired: 1 in, 1 out]
        }
        frame 1 {
          # "DATALOG OF OP 10"
          n553 = Enqueue Element(queue=w1484, element=cluster{"CASE 2":T12} {"CASE 2"=enum."SCAN1"}, error in (no error)=w1486) -> (queue out=w1483:refnum<queue>, error out=w1485:errorcluster)  [unwired: 1 in, 1 out]
        }
        frame 2 {
          # "SCAN BARCODE OP 20"
          n554 = Enqueue Element(queue=w1491, element=cluster{"CASE 2":T12} {"CASE 2"=enum."SCAN2"}, error in (no error)=w1490) -> (queue out=w1489:refnum<queue>, error out=w1488:errorcluster)  [unwired: 1 in, 1 out]
        }
        frame 3 {
          # "DATALOG OF OP 20"
          n555 = Enqueue Element(queue=w1496, element=cluster{"CASE 2":T12} {"CASE 2"=enum."DATALOG2"}, error in (no error)=w1495) -> (queue out=w1494:refnum<queue>, error out=w1493:errorcluster)  [unwired: 1 in, 1 out]
        }
        frame 4 {
          # "SCAN BARCODE OP 30"
          n556 = Enqueue Element(queue=w1501, element=cluster{"CASE 2":T12} {"CASE 2"=enum."SCAN3"}, error in (no error)=w1500) -> (queue out=w1499:refnum<queue>, error out=w1498:errorcluster)  [unwired: 1 in, 1 out]
        }
        frame 5 {
          # "DATALOG OF OP 30"
          n557 = Enqueue Element(queue=w1506, element=cluster{"CASE 2":T12} {"CASE 2"=enum."DATALOG3"}, error in (no error)=w1505) -> (queue out=w1504:refnum<queue>, error out=w1503:errorcluster)  [unwired: 1 in, 1 out]
        }
        frame 6 {
          # "SCAN BARCODE OP 40"
          n558 = Enqueue Element(queue=w1511, element=cluster{"CASE 2":T12} {"CASE 2"=enum."SCAN4"}, error in (no error)=w1510) -> (queue out=w1509:refnum<queue>, error out=w1508:errorcluster)  [unwired: 1 in, 1 out]
        }
        frame 7 {
          # "DATALOG OF OP 40"
          n559 = Enqueue Element(queue=w1516, element=cluster{"CASE 2":T12} {"CASE 2"=enum."DATALOG4"}, error in (no error)=w1515) -> (queue out=w1514:refnum<queue>, error out=w1513:errorcluster)  [unwired: 1 in, 1 out]
        }
        frame 8 {
          # "SCAN BARCODE OP 50"
          n560 = Enqueue Element(queue=w1521, element=cluster{"CASE":T12} {"CASE"=enum."SCAN5"}, error in (no error)=w1520) -> (queue out=w1519:refnum<queue>, error out=w1518:errorcluster)  [unwired: 1 in, 1 out]
        }
        frame 9 {
          # "DATALOG OF OP 50"
          n561 = Enqueue Element(queue=w1526, element=cluster{"CASE":T12} {"CASE"=enum."DATALOG5"}, error in (no error)=w1525) -> (queue out=w1524:refnum<queue>, error out=w1523:errorcluster)  [unwired: 1 in, 1 out]
        }
        frame 10 {
          # "SCAN BARCODE OP 60"
          n562 = Enqueue Element(queue=w1531, element=cluster{"CASE 2":T12} {"CASE 2"=enum."SCAN6"}, error in (no error)=w1530) -> (queue out=w1529:refnum<queue>, error out=w1528:errorcluster)  [unwired: 1 in, 1 out]
        }
        frame 11 {
          # "DATALOG OF OP 60"
          n563 = Enqueue Element(queue=w1536, element=cluster{"CASE 2":T12} {"CASE 2"=enum."DATALOG6"}, error in (no error)=w1535) -> (queue out=w1534:refnum<queue>, error out=w1533:errorcluster)  [unwired: 1 in, 1 out]
        }
        frame 12 {
          # "SCAN BARCODE OP 70"
          n564 = Enqueue Element(queue=w1541, element=cluster{"CASE 2":T12} {"CASE 2"=enum."SCAN7"}, error in (no error)=w1540) -> (queue out=w1539:refnum<queue>, error out=w1538:errorcluster)  [unwired: 1 in, 1 out]
        }
        frame 13 {
          # "DATALOG OF OP 70"
          n565 = Enqueue Element(queue=w1546, element=cluster{"CASE 2":T12} {"CASE 2"=enum."DATALOG7"}, error in (no error)=w1545) -> (queue out=w1544:refnum<queue>, error out=w1543:errorcluster)  [unwired: 1 in, 1 out]
        }
        frame 14 {
          # "SCAN BARCODE 80"
          n566 = Enqueue Element(queue=w1551, element=cluster{"CASE 2":T12} {"CASE 2"=enum."SCAN8"}, error in (no error)=w1550) -> (queue out=w1549:refnum<queue>, error out=w1548:errorcluster)  [unwired: 1 in, 1 out]
        }
        frame 15 {
          # "DATALOG OF OP 80"
          n567 = Enqueue Element(queue=w1556, element=cluster{"CASE 2":T12} {"CASE 2"=enum."DATALOG8"}, error in (no error)=w1555) -> (queue out=w1554:refnum<queue>, error out=w1553:errorcluster)  [unwired: 1 in, 1 out]
        }
        frame 16 {
          # "SCAN BARCODE OP 90"
          n568 = Enqueue Element(queue=w1561, element=cluster{"CASE 2":T12} {"CASE 2"=enum."SCAN9"}, error in (no error)=w1560) -> (queue out=w1559:refnum<queue>, error out=w1558:errorcluster)  [unwired: 1 in, 1 out]
        }
        frame 17 {
          # "DATALOG OF OP 90"
          n569 = Enqueue Element(queue=w1566, element=cluster{"CASE 2":T12} {"CASE 2"=enum."DATALOG9"}, error in (no error)=w1565) -> (queue out=w1564:refnum<queue>, error out=w1563:errorcluster)  [unwired: 1 in, 1 out]
        }
        frame 18 {
          # "SCAN BARCODE OP 100"
          n570 = Enqueue Element(queue=w1571, element=cluster{"CASE 2":T12} {"CASE 2"=enum."SCAN10"}, error in (no error)=w1570) -> (queue out=w1569:refnum<queue>, error out=w1568:errorcluster)  [unwired: 1 in, 1 out]
        }
        frame 19 {
          # "DATALOG OF OP 100"
          n571 = Enqueue Element(queue=w1576, element=cluster{"CASE 2":T12} {"CASE 2"=enum."DATALOG10"}, error in (no error)=w1575) -> (queue out=w1574:refnum<queue>, error out=w1573:errorcluster)  [unwired: 1 in, 1 out]
        }
        frame 20 {
          # "SCAN BARCODE OP 110"
          n572 = Enqueue Element(queue=w1581, element=cluster{"CASE 2":T12} {"CASE 2"=enum."SCAN11"}, error in (no error)=w1580) -> (queue out=w1579:refnum<queue>, error out=w1578:errorcluster)  [unwired: 1 in, 1 out]
        }
        frame 21 {
          # "DATALOG OF OP 110"
          n573 = Enqueue Element(queue=w1586, element=cluster{"CASE 2":T12} {"CASE 2"=enum."DATALOG11"}, error in (no error)=w1585) -> (queue out=w1584:refnum<queue>, error out=w1583:errorcluster)  [unwired: 1 in, 1 out]
        }
      }
    }
    n574 = Wait (ms)(milliseconds to wait=u32 50) -> ()  [unwired: 1 out]
    n575 = global read "Global 1.vi" "PLC COMM"() -> (→"PLC COM.":bool)
    n576 = global read "Global 1.vi" "PLC 1"() -> (→"OP 10 & 20":bool)
    n577 = global read "Global 1.vi" "PLC 2"() -> (→"OP 30":bool)
    n578 = global read "Global 1.vi" "PLC 3"() -> (→"OP 40":bool)
    n579 = case shown="False" "stop 2" {
      tunnel: w1425 -> [w1435 w1441]
      tunnel: [w1435 w1440] -> w1423
      tunnel: w1424 -> [w1434 w1439]
      tunnel: [w1434 w1438] -> w1422
      tunnel: [FALSE TRUE] -> w1421
      frame False {
      }
      frame True {
        n580 = Flush Queue(queue=w1441, error in (no error)=w1439) -> (queue out=w1443:refnum<queue>, error out=w1442:errorcluster)  [unwired: 1 out]
        n581 = Enqueue Element(queue=w1443, element=cluster{"CASE 2":T12} {"CASE 2"=enum."STOP"}, error in (no error)=w1442) -> (queue out=w1440:refnum<queue>, error out=w1438:errorcluster)  [unwired: 1 in, 1 out]
      }
    }
    "stop" <- w1421
    n582 = global read "Global 1.vi" "PLC 4"() -> (→"OP 50":bool)
    n583 = global read "Global 1.vi" "PLC 5"() -> (→"OP 60":bool)
    n584 = global read "Global 1.vi" "PLC 7"() -> (→"OP 90 -100 - 110":bool)
    n585 = global read "Global 1.vi" "PLC 6"() -> (→"OP 70 & 80":bool)
  }
  n586 = Release Queue(queue=w66, error in (no error)=w72) -> (error out=w49:errorcluster)  [unwired: 1 in, 2 out]
  n587 = call <vilib>:"Clear Errors.vi"("error in (no error)"=w68) -> ("error out"=w53:errorcluster)  [unwired: 5 in, 1 out]
  n588 = call <vilib>:"DB Tools Close Connection.vi"("error in (no error)"=w53, "connection reference"=w67) -> ("error out"=w50:errorcluster)  [unwired: 5 in]
  n589 = Merge Errors(w49, w50) -> (w51:errorcluster)
  n590 = call <vilib>:"Simple Error Handler.vi"("error in (no error)"=w51) -> ("error out"=w46:errorcluster)  [unwired: 4 in, 4 out]
  n591 = call <vilib>:"Clear Errors.vi"("error in (no error)"=w46) -> ("error out"=w52:errorcluster)  [unwired: 5 in, 1 out]
  n592 = flat-sequence {
    tunnel: w52 -> [w1589]
    tunnel: [w1589] -> w54
    frame #0 {
      n593 = global write "Global 1.vi" "REMOVE VI"(TRUE ("remove_VI")) -> ()
      n594 = global write "DATA LOG.vi" "Auto Cycle On"(FALSE) -> ()
    }
  }
  n595 = property class="App"(error in=w54) -> (error out=w56:errorcluster, "App.Kind"=w55:T36)  [unwired: 1 in, 1 out]
  n596 = case shown="\"Run Time System\"" w55 {
    tunnel: [w1590 w1592] -> w57
    tunnel: w56 -> [w1590 w1591]
    frame "Development System", Default {
    }
    frame "Run Time System" {
      n597 = invoke class="VI" method="FP.Close"(error in=w1591) -> (error out=w1592:errorcluster)  [unwired: 2 in, 2 out]
    }
  }
  "error out 2" <- w57
